vi "main.vi"() -> ()   [LabVIEW 2016]
uses:
  <userlib>/atmcd64d.llb/Error Code Enum typedef.ctl
  <userlib>/atmcd64d.llb/Shutter_mode typedef.ctl
  <vilib>/Utility/miscctls.llb/LVPoint32TypeDef.ctl
  <userlib>/atmcd64d.llb/Shutter_type typedef.ctl
  subVIs/variables/configDB.vi
  subVIs/variables/imageSettings.vi
  subVIs/variables/applicationControl.vi
  subVIs/variables/displayImage.vi
panel:
  in  "left profie location":dbl caption="Wavelength" step=1.0 format="%#.5f"
  in  "right Coords":T1
  in  "Read File":bool
  in  "Read mode":bool
  in  "right wvf scale 3":bool
  in  "left wvf scale 2":bool
  in  "right graph scale 2":bool
  in  "left graph scale":bool
  in  "right wvf color 4":u32(colorbox)=16725034 caption="Marker Color"
  in  "left wvf color 3":u32(colorbox)=16725034 caption="Marker Color"
  in  "left color 2":u32(colorbox)=16725034 caption="Marker Color"
  in  "right color":u32(colorbox)=16725034 caption="Marker Color"
  in  "graph real ratio?":bool caption="Fill screen / Real ratio"
  in  "left Coords":T1
  in  "line avg?":bool
  in  "Line Profile":string(combo)="Horizontal"
  out "scanned?":bool
  in  "right WaveMouse 2":i32
  in  "right Wavelength":dbl caption="Wavelength" step=1.0 format="%#.2f"
  out "Intensity 2":i32 caption="Intensity"
  out "right wvf graph":i32[](graph) caption="On Sensor Image Average"
  in  "left Wavelength":dbl caption="Y (mm)" step=0.01 format="%.2f"
  out "Intensity":i32
  in  "left WaveMouse":i32
  in  "Divide Reference":bool
  in  "Substract Background":bool
  in  "Reference":bool
  in  "Background":bool
  in  "ROI Scan":bool
  in  "ROI":cluster{dbl, dbl}(slide)={143.34131736526948, 408.85429141716565} scale=10.0..535.4
  out "OM":picture
  in  "Exposure Time":u16(ring)=128 items=["1/8000"=160, "1/6400"=157, "1/6000"=156, "1/5000"=155, "1/4000"=152, "1/3200"=149, "1/3000"=148, "1/2500"=147, "1/2000"=144, "1/1600"=141, "1/1500"=140, "1/1250"=139, "1/100"=136, "1/800"=133, "1/640"=131, "1/500"=128, "1/400"=125, "1/320"=123, "1/250"=120, "1/200"=117, "1/160"=115, "1/125"=112, "1/100"=109, "1/80"=107, "1/60"=104, "1/50"=101, "1/40"=99, "1/30"=96, "1/25"=93, "1/8"=80, "1/6"=77, "1/5"=75, "1/4"=72, "0\"3"=69, "0\"4"=67, "0\"5"=64, "0\"6"=61, "0\"7"=60, "0\"8"=59, "1\""=56, "1\"3"=53, "1\"5"=52, "1\"6"=51, "2\""=48, "2\"5"=45, "3\""=44, "3\"2"=43, "4\""=40, "5\""=37, "6\""=35, "8\""=32, "10\""=29, "13\""=27, "15\""=24, "20\""=21, "25\""=19, "30\""=16]
  in  "ISO":u32(ring) items=["Auto"=0, "50"=64, "100"=72, "125"=75, "160"=77, "200"=80, "250"=83, "320"=85, "400"=88, "500"=91, "640"=93, "800"=96, "1000"=99, "1250"=101, "1600"=104, "2000"=107, "2500"=109, "3200"=112, "4000"=115, "5000"=117, "6400"=120, "8000"=123, "10000"=125, "12800"=128, "25600"=136, "51200"=144, "102400"=152, "204800"=160, "409600"=168]
  out "Constructing data":i32(slide) scale=0.0..384.0
  out "Scanning done":bool
  in  "String":string
  in  "Exposure Time:":dbl(slide) scale=1.0..100.0
  out "ET Labelµ":dbl format="%#_3g"
  out "new picture":picture
  in  "Red Gain":i32(slide)=20 scale=1.0..64.0
  in  "Green Gain":i32(slide)=16 scale=1.0..64.0
  in  "Blue Gain":i32(slide)=17 scale=1.0..64.0
  in  "Gain?":bool
  in  "gamma":i32=10 min=1 max=20
  in  "contrast":i32=50 min=0 max=100
  in  "bright":i32=50 min=0 max=100
  in  "sharp":i32 min=0 max=3
  in  "OM":bool
  out "Moving":bool
  in  "Go Origin":bool caption="Origin Return"
  in  "Set Origin":bool
  in  "Stage Position":string
  out "Cooler":bool
  in  "Go back after scan":bool=TRUE
  in  "Scan Step (um)":dbl
  in  "Step length (um)":dbl=100.0
  in  "go left Button":bool
  in  "go right Button":bool
  in  "Y":dbl step=0.01 format="%#_3g"
  in  "X":dbl step=0.01 format="%#_3g"
  in  "Wipe and Quit":bool
  in  "Path":path=path "C:/Users/Administrator/Desktop/test"
  in  "Bandwidth (Frame)":dbl
  in  "Wavelength slide":i32(slide) scale=413.4192199707031..1005.0010375976562
  out "left wvf graph":i32[](graph) caption="On Sensor Image Average"
  out "Right Graph":i32[][](graph) caption="Object Image"
  out "Recovering Temperature":bool
  out "Left Graph":i32[][](graph) caption="On Sensor Image"
  out "temp. status 2":T2
  out "Detector Model":string
  in  "Save File":bool
  in  "Shut Down":bool
  in  "Scan Abort":bool
  out "Current \nScan Frame":dbl
  out "Total \nScan Frame":dbl
  in  "Scan Start":bool
  in  "Scan Length (mm)":dbl=25.0
  in  "Shutter Control":T3=enum."Close"
  in  "Exposure Time (s)":sgl=0.01 step=0.001 format="%.4f"
  in  "Take shot":bool
  in  "VSS (s)":u16(ring)
  in  "HSS (MHz)":i32(ring)
  in  "Live View":bool
  out "Status":T2
  out "Temperature":dbl
  in  "Set Temperature":dbl=20.0
  in  "Initilization File":path=path "C:/Users/Administrator/Desktop/micro.ini"
  # "Image Settings"
  # "Stage Control"
  # "File"
  # "Scan"
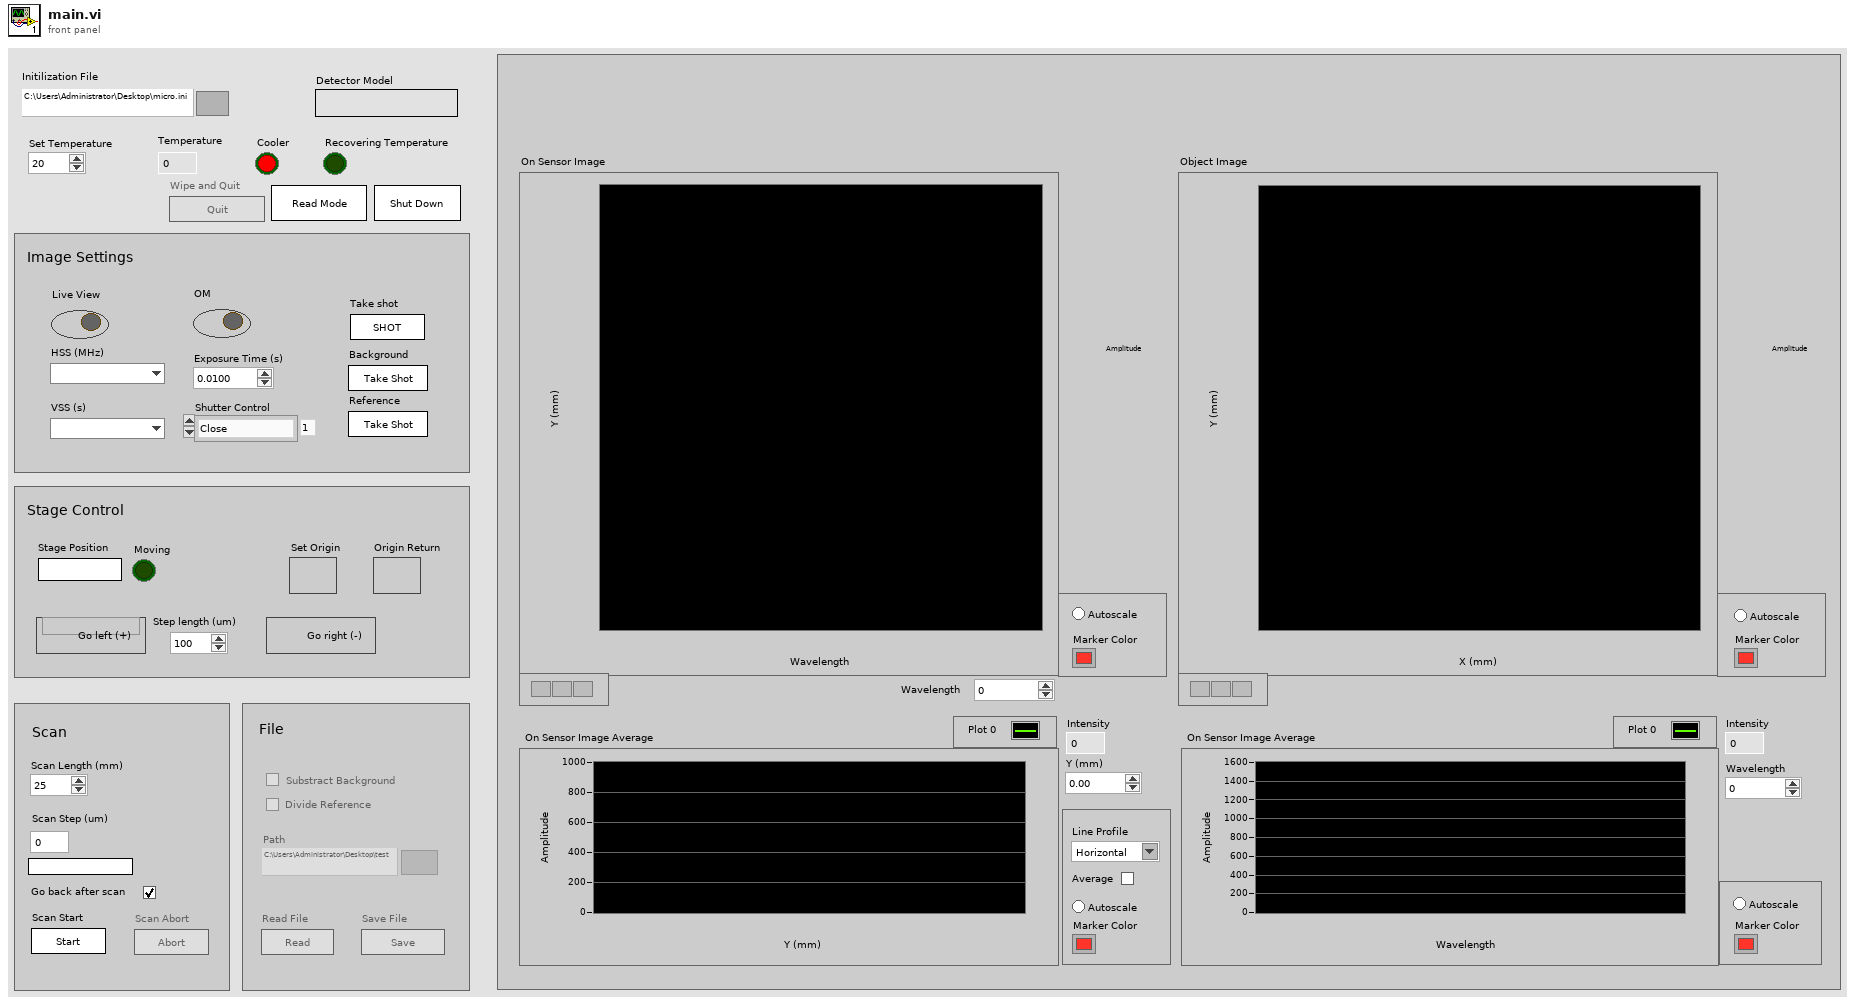
[diagram p1: front panel]
types:
  T1 = typedef "LVPoint32TypeDef.ctl" = cluster{"Horizontal":i32, "Vertical":i32}
  T2 = typedef "Error Code Enum typedef.ctl" = enum32{"N/A (0)", "DRV_ERROR_CODES", "DRV_SUCCESS", "DRV_VXDNOTINSTALLED", "DRV_ERROR_SCAN", "DRV_ERROR_CHECK_SUM", "DRV_ERROR_FILELOAD", "DRV_UNKNOWN_FUNC", "DRV_ERROR_VXD_INIT", "DRV_ERROR_ADDRESS", "DRV_ERROR_PAGELOCK", "DRV_ERROR_PAGEUNLOCK", "DRV_ERROR_BOARDTEST", "DRV_ERROR_ACK", "DRV_ERROR_UP_FIFO", "DRV_ERROR_PATTERN", "N/A (16)", "DRV_ACQUISITION_ERRORS", "DRV_ACQ_BUFFER", "DRV_ACQ_DOWNFIFO_FULL", "DRV_PROC_UNKONWN_INSTRUCTION", "DRV_ILLEGAL_OP_CODE", "DRV_KINETIC_TIME_NOT_MET", "DRV_ACCUM_TIME_NOT_MET", "DRV_NO_NEW_DATA", "N/A (25)", "DRV_SPOOLERROR", "N/A (27)", "N/A (28)", "N/A (29)", "N/A (30)", "N/A (31)", "N/A (32)", "DRV_TEMPERATURE_CODES", "DRV_TEMPERATURE_OFF", "DRV_TEMPERATURE_NOT_STABILIZED", "DRV_TEMPERATURE_STABILIZED", "DRV_TEMPERATURE_NOT_REACHED", "DRV_TEMPERATURE_OUT_RANGE", "DRV_TEMPERATURE_NOT_SUPPORTED", "DRV_TEMPERATURE_DRIFT", "N/A (41)", "N/A (42)", "N/A (43)", "N/A (44)", "N/A (45)", "N/A (46)", "N/A (47)", "N/A (48)", "DRV_GENERAL_ERRORS", "DRV_INVALID_AUX", "DRV_COF_NOTLOADED", "DRV_FPGAPROG", "DRV_FLEXERROR", "DRV_GPIBERROR", "N/A (55)", "N/A (56)", "N/A (57)", "N/A (58)", "N/A (59)", "N/A (60)", "N/A (61)", "N/A (62)", "N/A (63)", "DRV_DATATYPE", "DRV_DRIVER_ERRORS", "DRV_P1INVALID", "DRV_P2INVALID", "DRV_P3INVALID", "DRV_P4INVALID", "DRV_INIERROR", "DRV_COFERROR", "DRV_ACQUIRING", "DRV_IDLE", "DRV_TEMPCYCLE", "DRV_NOT_INITIALIZED", "DRV_P5INVALID", "DRV_P6INVALID", "DRV_INVALID_MODE", "DRV_INVALID_FILTER", "DRV_I2CERRORS", "DRV_I2CDEVNOTFOUND", "DRV_I2CTIMEOUT", "DRV_P7INVALID", "N/A (84)", "N/A (85)", "N/A (86)", "N/A (87)", "N/A (88)", "N/A (89)", "DRV_IOCERROR", "DRV_VRMVERSIONERROR"}
  T3 = typedef "Shutter_mode typedef.ctl" = enum16{"Auto", "Close", "Open", "N/A (3)", "Open FVB Series", "Open Any Series"}
  T4 = enum8{"Enabled", "Disabled", "Disabled and Grayed Out"}
  T5 = cluster{"Width":u16, "Style":enum32{"Solid", "Dash", "Dot", "DashDot", "DashDotDot"}}
  T6 = typedef "Shutter_type typedef.ctl" = enum16{"TTL Low", "TTL High"}
  T7 = typedef "HSSpeed_type typedef.ctl" = enum16{"EM Amp", "Conventional Amp"}
  T8 = typedef "LVMouseTypeDef.ctl" = cluster{"Mouse Position":cluster{"X":i32, "Y":i32}, "Mouse Modifiers":cluster{"Button Down":bool, "Shift Mod":bool, "Menu Mod":bool, "Option Mod":bool}}
  T9 = typedef "imagedata.ctl" = cluster{"image type":i32, "image depth":i32, "image":u8[], "mask":u8[], "colors":u32[], "Rectangle":cluster{"left":i16, "top":i16, "right":i16, "bottom":i16}}
  T10 = typedef "LVBoundsTypeDef.ctl" = cluster{"Width":u32, "Height":u32}
  T11 = cluster{"left":i16, "top":i16, "right":i16, "bottom":i16}
  T12 = cluster{"Scan Abort":refnum<vi>, "Constructing data":refnum<vi>, "Right Graph":refnum<vi>, "Left Graph":refnum<vi>, "Total \nScan Frame":refnum<vi>, "Current \nScan Frame":refnum<vi>}
  T13 = typedef "LVRectTypeDef.ctl" = cluster{"Left":i16, "Top":i16, "Right":i16, "Bottom":i16}
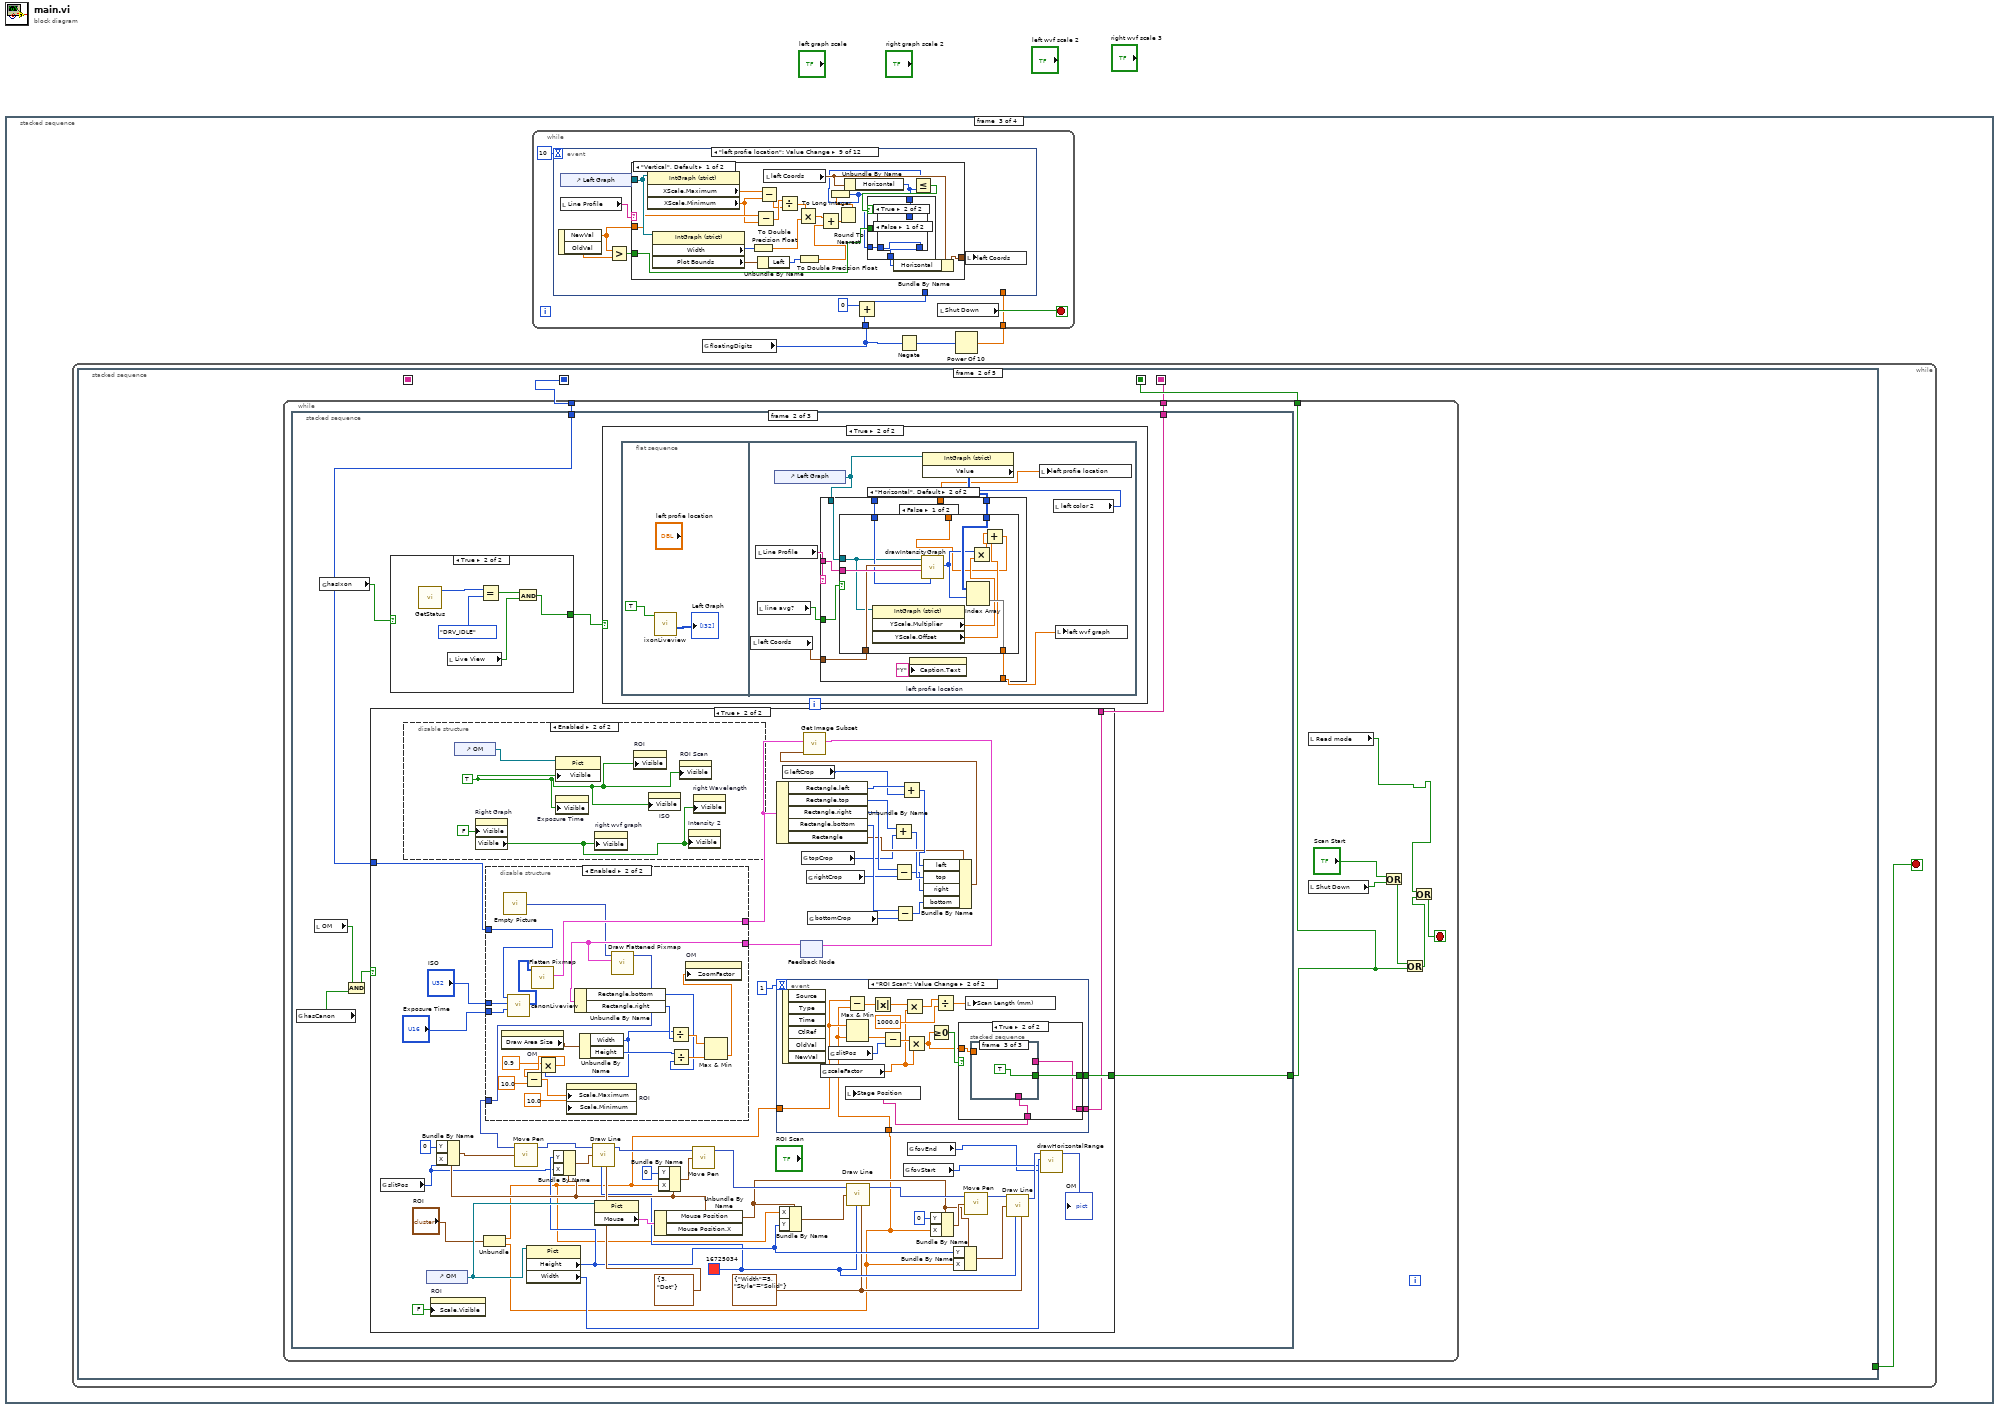
[diagram p0: block diagram]
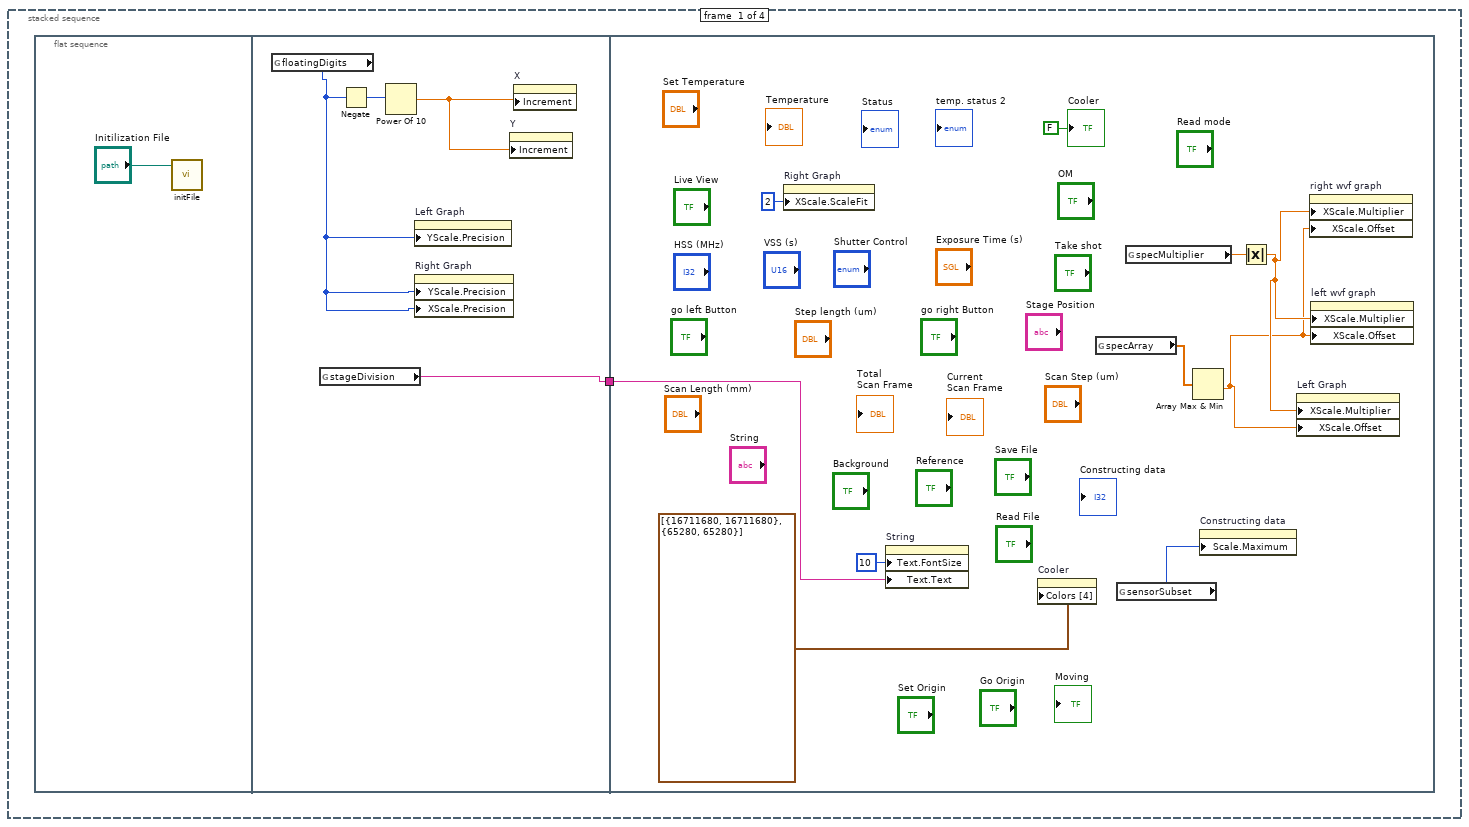
[diagram p2: hidden frame]
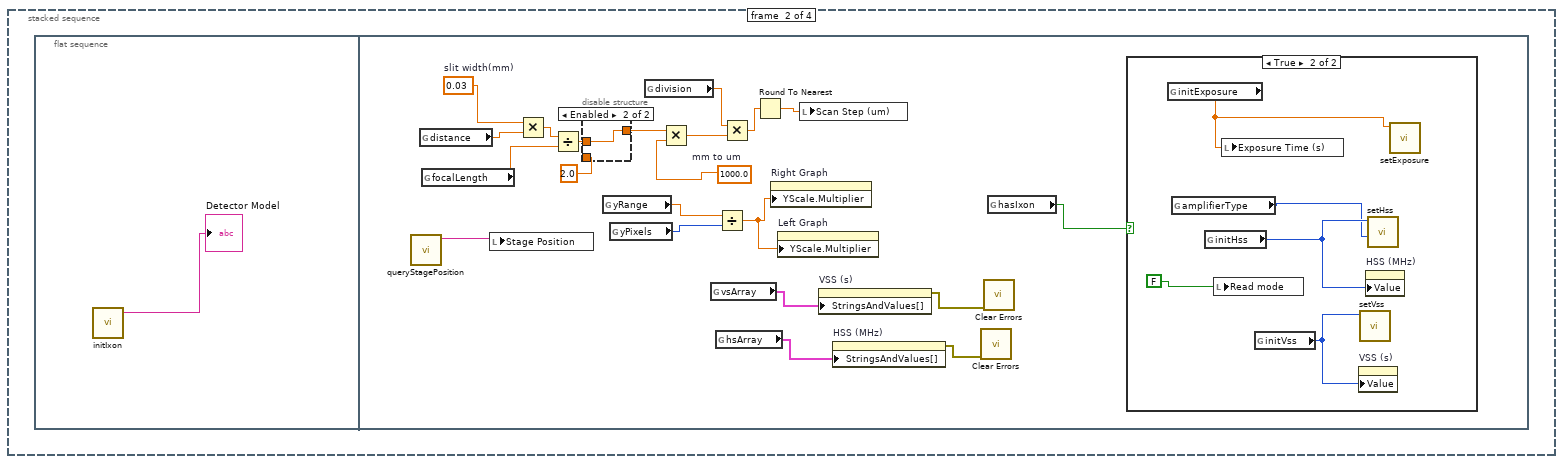
[diagram p3: hidden frame]
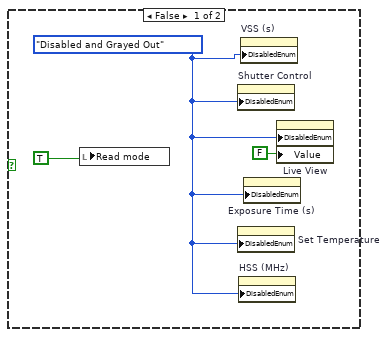
[diagram p4: hidden frame]
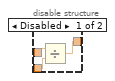
[diagram p5: hidden frame]
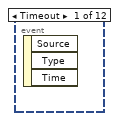
[diagram p6: hidden frame]
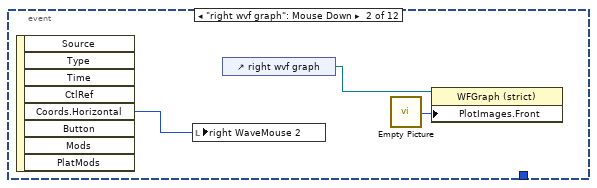
[diagram p7: hidden frame]
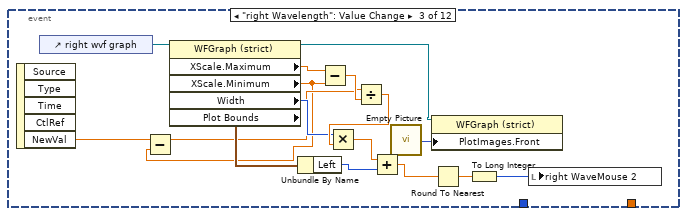
[diagram p8: hidden frame]
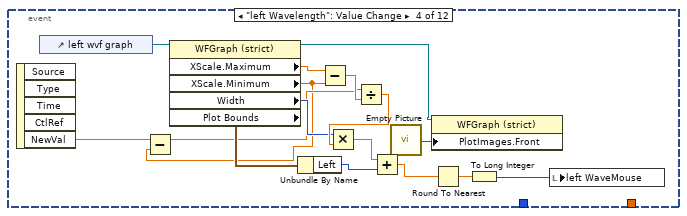
[diagram p9: hidden frame]
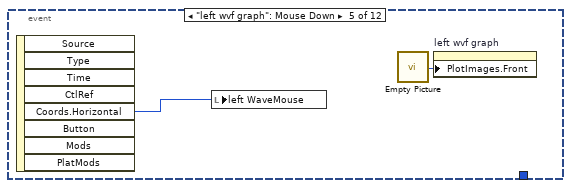
[diagram p10: hidden frame]
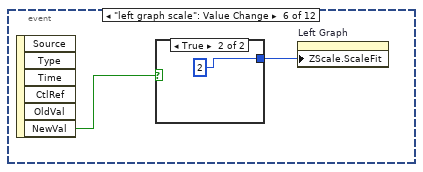
[diagram p11: hidden frame]
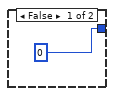
[diagram p12: hidden frame]
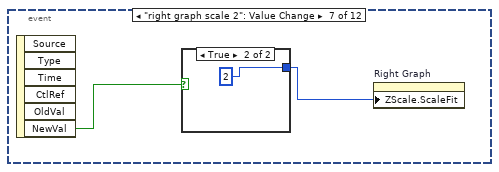
[diagram p13: hidden frame]
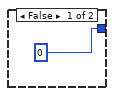
[diagram p14: hidden frame]
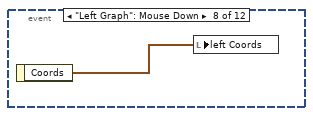
[diagram p15: hidden frame]
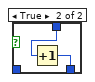
[diagram p17: hidden frame]
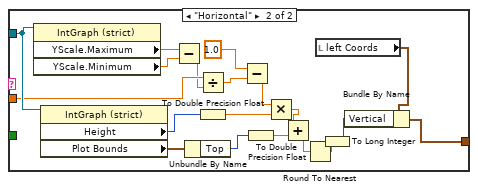
[diagram p18: hidden frame]
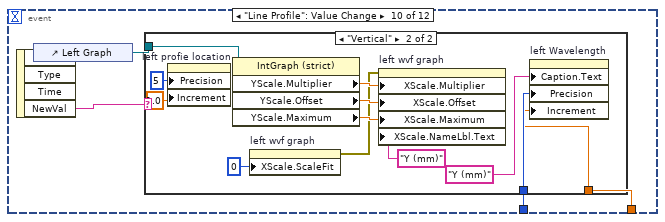
[diagram p19: hidden frame]
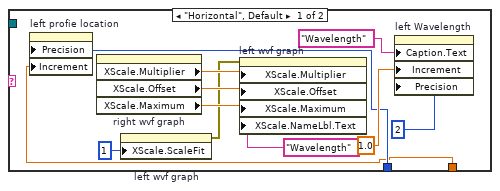
[diagram p20: hidden frame]
diagram:
  n1 = stacked-sequence {
    frame #0 {
      n2 = flat-sequence {
        tunnel: [w6] -> w1
        tunnel: w1 -> [w13]
        frame #0 {
          n3 = call "initFile.vi"("Init File"="Initilization File") -> ()  [unwired: 11 in]
        }
        frame #1 {
          n4 = global read "configDB.vi" "floatingDigits"() -> (w5:i32)
          n5 = global read "configDB.vi" "stageDivision"() -> (w6:string)
          n6 = Negate(x=w5) -> (-x=w4:i32)
          n7 = Power Of 10(x=w4) -> (10^x=w3:dbl)
          n8 = property on="Left Graph" class="IntGraph (strict)"("YScale.Precision"=w5) -> ()  [unwired: 2 in, 2 out]
          n9 = property on="Right Graph" class="IntGraph (strict)"("YScale.Precision"=w5, "XScale.Precision"=w5) -> ()  [unwired: 2 in, 2 out]
          n10 = property on="Y" class="DigNum (strict)"("Increment"=w3) -> ()  [unwired: 2 in, 2 out]
          n11 = property on="X" class="DigNum (strict)"("Increment"=w3) -> ()  [unwired: 2 in, 2 out]
        }
        frame #2 {
          n12 = property on="Right Graph" class="IntGraph (strict)"("XScale.ScaleFit"=u8 2 ("X Scale.Scale Fit")) -> ()  [unwired: 2 in, 2 out]
          n13 = property on="String" class="Str"("Text.FontSize"=u32 10 ("Text.Font:Size"), "Text.Text"=w13) -> ()  [unwired: 2 in, 2 out]
          n14 = property on="Cooler" class="Bool (strict)"("Colors [4]"=cluster{u32, u32}[] [{16711680, 16711680}, {65280, 65280}]) -> ()  [unwired: 2 in, 2 out]
          n15 = global read "imageSettings.vi" "specArray"() -> (w10:sgl[])
          n16 = global read "configDB.vi" "sensorSubset"() -> (w7:i32)
          n17 = global read "configDB.vi" "specMultiplier"() -> (w11:dbl)
          n18 = Array Max & Min(array=w10) -> (min value=w8:sgl)  [unwired: 3 out]
          n19 = property on="Constructing data" class="Slide (strict)"("Scale.Maximum"=w7) -> ()  [unwired: 2 in, 2 out]
          n20 = Absolute Value(x=w11) -> (abs(x)=w9:dbl)
          n21 = property on="Left Graph" class="IntGraph (strict)"("XScale.Multiplier"=w9, "XScale.Offset"=w8) -> ()  [unwired: 2 in, 2 out]
          n22 = property on="right wvf graph" class="WFGraph (strict)"("XScale.Multiplier"=w9, "XScale.Offset"=w8) -> ()  [unwired: 2 in, 2 out]
          n23 = property on="left wvf graph" class="WFGraph (strict)"("XScale.Multiplier"=w9, "XScale.Offset"=w8) -> ()  [unwired: 2 in, 2 out]
          "Cooler" <- FALSE ("Cooler")
        }
      }
    }
    frame #1 {
      n24 = flat-sequence {
        frame #0 {
          n25 = call "initIxon.vi"() -> ("model"=→"Detector Model":string)  [unwired: 5 in, 2 out]
        }
        frame #1 {
          w30 = 1000.0  # mm to um
          w37 = 0.03  # slit width(mm)
          n26 = call "queryStagePosition.vi"() -> ("stagePosition"=w28:string)  [unwired: 11 in]
          n27 = global read "configDB.vi" "distance"() -> (w26:dbl)
          n28 = global read "configDB.vi" "focalLength"() -> (w25:dbl)
          n29 = local write "Stage Position"(w28) -> ()
          n30 = Multiply(x=w37, y=w26) -> (x*y=w36:dbl)
          n31 = Divide(x=w36, y=w25) -> (x/y=w34:dbl)
          n32 = disable-structure shown="Enabled" {
            disable-tunnel: w34 -> [w49 w50]
            disable-tunnel: 2.0 ("y") -> [w48 _]
            disable-tunnel: [w47 w50] -> w32
            frame Disabled {
              n33 = Divide(x=w49, y=w48) -> (x/y=w47:dbl)
            }
            frame Enabled {
            }
          }
          n34 = global read "configDB.vi" "yRange"() -> (w24:dbl)
          n35 = global read "configDB.vi" "yPixels"() -> (w19:i32)
          n36 = global read "configDB.vi" "division"() -> (w27:dbl)
          n37 = Multiply(x=w32, y=w30) -> (x*y=w35:dbl)
          n38 = global read "imageSettings.vi" "vsArray"() -> (w22:cluster{"String":string, "Value":u16}[])
          n39 = global read "imageSettings.vi" "hsArray"() -> (w23:cluster{"String":string, "Value":u16}[])
          n40 = Divide(x=w24, y=w19) -> (x/y=w38:dbl)
          n41 = Multiply(x=w27, y=w35) -> (x*y=w31:dbl)
          n42 = Round To Nearest(number=w31) -> (nearest integer value=w29:dbl)
          n43 = property on="Right Graph" class="IntGraph (strict)"("YScale.Multiplier"=w38) -> ()  [unwired: 2 in, 2 out]
          n44 = property on="Left Graph" class="IntGraph (strict)"("YScale.Multiplier"=w38) -> ()  [unwired: 2 in, 2 out]
          n45 = local write "Scan Step (um)"(w29) -> ()
          n46 = property on="VSS (s)" class="Ring (strict)"("StringsAndValues[]"=w22) -> (error out=w21:errorcluster)  [unwired: 2 in, 1 out]
          n47 = property on="HSS (MHz)" class="Ring (strict)"("StringsAndValues[]"=w23) -> (error out=w20:errorcluster)  [unwired: 2 in, 1 out]
          n48 = call <vilib>:"Clear Errors.vi"("error in (no error)"=w20) -> ()  [unwired: 5 in, 2 out]
          n49 = call <vilib>:"Clear Errors.vi"("error in (no error)"=w21) -> ()  [unwired: 5 in, 2 out]
          n50 = global read "applicationControl.vi" "hasIxon"() -> (w18:bool)
          n51 = case shown="True" w18 {
            frame False {
              w41 = T4."Disabled and Grayed Out" ("Disabled")
              n52 = local write "Read mode"(TRUE) -> ()
              n53 = property on="Shutter Control" class="Enum (strict)"("DisabledEnum"=w41) -> ()  [unwired: 2 in, 2 out]
              n54 = property on="Set Temperature" class="DigNum (strict)"("DisabledEnum"=w41) -> ()  [unwired: 2 in, 2 out]
              n55 = property on="HSS (MHz)" class="Ring (strict)"("DisabledEnum"=w41) -> ()  [unwired: 2 in, 2 out]
              n56 = property on="VSS (s)" class="Ring (strict)"("DisabledEnum"=w41) -> ()  [unwired: 2 in, 2 out]
              n57 = property on="Exposure Time (s)" class="DigNum (strict)"("DisabledEnum"=w41) -> ()  [unwired: 2 in, 2 out]
              n58 = property on="Live View" class="Bool (strict)"("DisabledEnum"=w41, "Value"=FALSE ("Live View")) -> ()  [unwired: 2 in, 2 out]
            }
            frame True {
              n59 = global read "configDB.vi" "initExposure"() -> (w46:dbl)
              n60 = global read "configDB.vi" "amplifierType"() -> (w43:T7)
              n61 = global read "configDB.vi" "initHss"() -> (w45:i32)
              n62 = local write "Read mode"(FALSE) -> ()
              n63 = local write "Exposure Time (s)"(w46) -> ()
              n64 = global read "configDB.vi" "initVss"() -> (w44:i32)
              n65 = property on="VSS (s)" class="Ring (strict)"("Value"=w44) -> ()  [unwired: 2 in, 2 out]
              n66 = call "setVss.vi"("index"=w44) -> ()  [unwired: 11 in]
              n67 = property on="HSS (MHz)" class="Ring (strict)"("Value"=w45) -> ()  [unwired: 2 in, 2 out]
              n68 = call "setHss.vi"("type"=w43, "index"=w45) -> ()  [unwired: 10 in]
              n69 = call "setExposure.vi"("Exposure Time (s)"=w46) -> ()  [unwired: 11 in]
            }
          }
        }
      }
    }
    frame #2 {
      n70 = while {
        stop <- w196 stop-if-true
        n71 = stacked-sequence {
          seq-local: [_ _ w535 _ _] -> [_ _ _ w565 _]
          seq-local: [w199 _ _ _ _] -> [_ w213 w534 _ _]
          seq-local: [_ w212 _ _ _] -> [_ _ _ w567 _]
          seq-local: [_ w211 _ _ _] -> [_ _ _ w566 _]
          tunnel: [_ _ _ _ w603] -> w196
          frame #0 {
            n72 = flat-sequence {
              tunnel: [w202] -> w199
              tunnel: [w201] -> w197
              tunnel: [w206] -> w198
              tunnel: w197 -> [w206]
              tunnel: w198 -> [w210]
              frame #0 {
                n73 = disable-structure shown="Enabled" {
                  disable-tunnel: [_ w205] -> w202
                  disable-tunnel: [_ w204] -> w201
                  frame Disabled {
                    n74 = call "initMightex.vi"() -> ()  [unwired: 11 in, 1 out]
                  }
                  frame Enabled {
                    n75 = call "initCanon.vi"() -> ("error out"=w203:errorcluster, "inRef dup"=w205:u32)  [unwired: 10 in]
                    n76 = Unbundle By Name(w203) -> ("status"=w204:bool)
                    n77 = call <vilib>:"Clear Errors.vi"("error in (no error)"=w203) -> ()  [unwired: 5 in, 2 out]
                  }
                }
              }
              frame #1 {
                n78 = global read "applicationControl.vi" "hasCanon"() -> (w207:bool)
                n79 = case shown="False" w207 {
                  frame False {
                    n80 = property on="OM" class="Bool (strict)"("DisabledEnum"=T4."Disabled and Grayed Out" ("Disabled"), "Value"=FALSE ("OM")) -> ()  [unwired: 2 in, 2 out]
                  }
                  frame True {
                  }
                }
              }
              frame #2 {
                n81 = case shown="True" w210 {
                  frame False {
                  }
                  frame True {
                    n82 = call "Display Message to User"() -> ()  [unwired: 10 in, 2 out]
                  }
                }
              }
            }
            n83 = call "queryStagePosition.vi"() -> ("stagePosition"=w200:string)  [unwired: 11 in]
            n84 = local write "Stage Position"(w200) -> ()
          }
          frame #1 {
            n85 = while {
              tunnel: w213 -> [w220]
              tunnel: [w218] -> w212
              tunnel: [w217] -> w211
              stop <- w215 stop-if-true
              n86 = stacked-sequence {
                tunnel: w220 -> [_ w288 _]
                tunnel: [_ w287 _] -> w218
                tunnel: [_ w286 _] -> w217
                frame #0 {
                  n87 = event shown="[3] \"Background\": Value Change" {
                    selector: _ -> [_ _ _ _ _ _ _ _ _ _ _ _ _ _]
                    dyn-events: _ -> [_ _ _ _ _ _ _ _ _ _ _ _ _ _]
                    timeout: 0 -> [_ _ _ _ _ _ _ _ _ _ _ _ _ _]
                    event "HSS (MHz)": Value Change {
                      n88 = event-data() -> ()  [unwired: 1 in, 6 out]
                      n89 = global read "configDB.vi" "amplifierType"() -> (w227:T7)
                      n90 = property on="HSS (MHz)" class="Ring (strict)"() -> ("Value"=w228:i32)  [unwired: 2 in, 2 out]
                      n91 = call "setHss.vi"("type"=w227, "index"=w228) -> ()  [unwired: 10 in]
                    }
                    event "VSS (s)": Value Change {
                      n92 = event-data() -> ()  [unwired: 1 in, 6 out]
                      n93 = property on="VSS (s)" class="Ring (strict)"() -> ("Value"=w229:u16)  [unwired: 2 in, 2 out]
                      n94 = call "setVss.vi"("index"=w229) -> ()  [unwired: 11 in]
                    }
                    event "Take shot": Value Change {
                      n95 = event-data() -> ()  [unwired: 1 in, 6 out]
                      n96 = flat-sequence {
                        frame #0 {
                          n97 = global read "configDB.vi" "specMultiplier"() -> (w233:dbl)
                          n98 = global read "imageSettings.vi" "specArray"() -> (w231:sgl[])
                          n99 = Array Max & Min(array=w231) -> (min value=w230:sgl)  [unwired: 3 out]
                          n100 = Absolute Value(x=w233) -> (abs(x)=w232:dbl)
                          n101 = property on="Right Graph" class="IntGraph (strict)"("XScale.Multiplier"=w232, "XScale.Offset"=w230, "XScale.NameLbl.Text"="Wavelength (nm)" ("X Scale.Name Label.Text"), "Caption.Text"="On Sensor Image" ("Label.Text")) -> ()  [unwired: 2 in, 2 out]
                        }
                        frame #1 {
                          n102 = call "ixonLiveview.vi"("stop"=TRUE) -> ("Left Graph"=→"Right Graph":i32[][])  [unwired: 10 in]
                        }
                        frame #2 {
                          n103 = control-ref of="Right Graph"() -> (w239:refnum<vi>)
                          n104 = property on="Property Node" class="IntGraph (strict)"(reference=w239) -> ("Value"=w238:i32[][])  [unwired: 1 in, 2 out]
                          n105 = for {
                            N: 384 -> [_]
                            tunnel: w238 -> [w247]
                            tunnel: [w242] -> w241 mode=indexing
                            i -> [w246]
                            n106 = Index Array(array=w247, index (col)=w246) -> (element=w245:i32[])  [unwired: 1 in]
                            n107 = Add Array Elements(numeric array=w245) -> (sum=w244:i32)
                            n108 = Divide(x=w244, y=512) -> (x/y=w242:dbl)
                          }
                          n109 = local write "right wvf graph"(w241) -> ()
                        }
                      }
                    }
                    event "Background": Value Change {
                      n110 = event-data() -> ()  [unwired: 1 in, 6 out]
                      n111 = flat-sequence {
                        frame #0 {
                          n112 = call "setShutterMode.vi"("mode"=Shutter_mode_typedef."Close") -> ()  [unwired: 11 in]
                        }
                        frame #1 {
                          n113 = Wait (ms)(milliseconds to wait=u32 1000) -> ()  [unwired: 1 out]
                        }
                        frame #2 {
                          n114 = call "ixonLiveview.vi"("stop"=TRUE) -> ("Left Graph"=w250:i32[][])  [unwired: 10 in]
                          n115 = global write "imageSettings.vi" "backgroundExist"(TRUE ("backgroundExist")) -> ()
                          n116 = local write "Right Graph"(w250) -> ()
                          n117 = call "background.vi"("Enum"=enum16{"clear", "read", "write"}."write", "backgroundImageIn"=w250) -> ()  [unwired: 9 in, 1 out]
                        }
                        frame #3 {
                          n118 = local read "Shutter Control"() -> (w254:T3)
                          n119 = call "setShutterMode.vi"("mode"=w254) -> ()  [unwired: 11 in]
                        }
                      }
                    }
                    event "Reference": Value Change {
                      n120 = event-data() -> ()  [unwired: 1 in, 6 out]
                      n121 = flat-sequence {
                        frame #0 {
                          n122 = call "setShutterMode.vi"("mode"=Shutter_mode_typedef."Open") -> ()  [unwired: 11 in]
                        }
                        frame #1 {
                          n123 = Wait (ms)(milliseconds to wait=u32 1000) -> ()  [unwired: 1 out]
                        }
                        frame #2 {
                          n124 = call "ixonLiveview.vi"("stop"=TRUE) -> ("Left Graph"=w257:i32[][])  [unwired: 10 in]
                          n125 = local write "Right Graph"(w257) -> ()
                          n126 = global write "imageSettings.vi" "referenceExist"(TRUE ("backgroundExist")) -> ()
                          n127 = call "reference.vi"("Enum"=enum16{"clear", "read", "write"}."write", "referenceImageIn"=w257) -> ()  [unwired: 9 in, 1 out]
                        }
                        frame #3 {
                          n128 = local read "Shutter Control"() -> (w261:T3)
                          n129 = call "setShutterMode.vi"("mode"=w261) -> ()  [unwired: 11 in]
                        }
                      }
                    }
                    event "go right Button": Value Change {
                      n130 = event-data() -> ()  [unwired: 1 in, 6 out]
                      n131 = flat-sequence {
                        frame #0 {
                          n132 = local write "Moving"(TRUE ("Moving")) -> ()
                        }
                        frame #1 {
                          n133 = local read "Step length (um)"() -> (w264:dbl)
                          n134 = call "stageGoRight.vi"("Step length (um)"=w264) -> ("Stage Position"=w263:string)  [unwired: 10 in]
                          n135 = local write "Stage Position"(w263) -> ()
                        }
                        frame #2 {
                          n136 = local write "Moving"(FALSE ("Moving")) -> ()
                        }
                      }
                    }
                    event "Go Origin": Value Change {
                      n137 = event-data() -> ()  [unwired: 1 in, 6 out]
                      n138 = flat-sequence {
                        frame #0 {
                          n139 = local write "Moving"(TRUE ("Moving")) -> ()
                        }
                        frame #1 {
                          n140 = call "stageGoOrigin.vi"() -> ()  [unwired: 12 in]
                        }
                        frame #2 {
                          n141 = local write "Stage Position"("0" ("Stage Position")) -> ()
                          n142 = local write "Moving"(FALSE ("Moving")) -> ()
                        }
                      }
                    }
                    event "Set Origin": Value Change {
                      n143 = event-data() -> ()  [unwired: 1 in, 6 out]
                      n144 = local write "Stage Position"("0" ("Stage Position")) -> ()
                      n145 = call "stageSetOrigin.vi"() -> ()  [unwired: 12 in]
                    }
                    event "go left Button": Value Change {
                      n146 = event-data() -> ()  [unwired: 1 in, 6 out]
                      n147 = flat-sequence {
                        frame #0 {
                          n148 = local write "Moving"(TRUE ("Moving")) -> ()
                        }
                        frame #1 {
                          n149 = local read "Step length (um)"() -> (w272:dbl)
                          n150 = call "stageGoLeft.vi"("Step length (um)"=w272) -> ("Stage Position"=w271:string)  [unwired: 10 in]
                          n151 = local write "Stage Position"(w271) -> ()
                        }
                        frame #2 {
                          n152 = local write "Moving"(FALSE ("Moving")) -> ()
                        }
                      }
                    }
                    event "Scan Step (um)": Value Change {
                      n153 = event-data() -> ()  [unwired: 1 in, 6 out]
                      n154 = local read "Scan Step (um)"() -> (w275:dbl)
                      n155 = global read "configDB.vi" "division"() -> (w274:dbl)
                      n156 = Quotient & Remainder(x=w275, y=w274) -> (x-y*floor(x/y)=w278:dbl)  [unwired: 1 out]
                      n157 = Equal?(x=w278, y=0.0) -> (x = y?=w276:bool)
                      n158 = case shown="False" w276 {
                        frame False {
                          n159 = call "Step too small!"() -> ()  [unwired: 18 in, 2 out]
                        }
                        frame True {
                        }
                      }
                    }
                    event Timeout {
                      n160 = event-data() -> ()  [unwired: 1 in, 3 out]
                    }
                    event Value Change {
                      n161 = event-data() -> ()  [unwired: 1 in, 6 out]
                      n162 = property on="Shutter Control" class="Enum (strict)"() -> ("Value"=w279:T3)  [unwired: 2 in, 2 out]
                      n163 = call "setShutterMode.vi"("mode"=w279) -> ()  [unwired: 11 in]
                    }
                    event "Exposure Time (s)": Value Change {
                      n164 = event-data() -> ()  [unwired: 1 in, 6 out]
                      n165 = local read "Exposure Time (s)"() -> (w280:sgl)
                      n166 = call "setExposure.vi"("Exposure Time (s)"=w280) -> ()  [unwired: 11 in]
                    }
                    event "Set Temperature": Value Change {
                      n167 = event-data() -> ()  [unwired: 1 in, 6 out]
                      n168 = local read "Set Temperature"() -> (w281:dbl)
                      n169 = call "setTemp.vi"("Set Temp."=w281) -> ()  [unwired: 11 in]
                    }
                  }
                  n170 = global read "imageSettings.vi" "backgroundExist"() -> (w223:bool)
                  n171 = case shown="True" w223 {
                    frame False {
                      n172 = property on="Reference" class="Bool"("DisabledEnum"=T4."Disabled and Grayed Out" ("Disabled")) -> ()  [unwired: 2 in, 2 out]
                    }
                    frame True {
                      n173 = property on="Reference" class="Bool"("DisabledEnum"=T4."Enabled" ("Disabled")) -> ()  [unwired: 2 in, 2 out]
                    }
                  }
                }
                frame #1 {
                  n174 = global read "applicationControl.vi" "hasCanon"() -> (w283:bool)
                  n175 = local read "OM"() -> (w284:bool)
                  n176 = global read "applicationControl.vi" "hasIxon"() -> (w282:bool)
                  n177 = And(x=w284, y=w283) -> (x .and. y?=w285:bool)
                  n178 = case shown="True" w285 {
                    tunnel: w288 -> [_ w432]
                    tunnel: [FALSE w389] -> w287
                    tunnel: [_ w385] -> w286
                    frame False {
                      w373 = FALSE ("Visible")
                      w377 = FALSE ("Visible")
                      n179 = property on="new picture" class="Pict"("Visible"=w377) -> ()  [unwired: 2 in, 2 out]
                      n180 = property on="sharp" class="DigNum (strict)"("Visible"=w377) -> ()  [unwired: 2 in, 2 out]
                      n181 = property on="bright" class="DigNum (strict)"("Visible"=w377) -> ()  [unwired: 2 in, 2 out]
                      n182 = property on="gamma" class="DigNum (strict)"("Visible"=w377) -> ()  [unwired: 2 in, 2 out]
                      n183 = property on="Exposure Time:" class="Slide (strict)"("Visible"=w377) -> ()  [unwired: 2 in, 2 out]
                      n184 = property on="ET Labelµ" class="DigNum (strict)"("Visible"=w377) -> ()  [unwired: 2 in, 2 out]
                      n185 = property on="Right Graph" class="IntGraph (strict)"("Visible"=TRUE) -> ("Visible"=w370:bool)  [unwired: 2 in, 2 out]
                      n186 = property on="right wvf graph" class="WFGraph (strict)"("Visible"=w370) -> ()  [unwired: 2 in, 2 out]
                      n187 = property on="right Wavelength" class="DigNum (strict)"("Visible"=w370) -> ()  [unwired: 2 in, 2 out]
                      n188 = property on="Intensity 2" class="DigNum (strict)"("Visible"=w370) -> ()  [unwired: 2 in, 2 out]
                      n189 = property on="contrast" class="DigNum (strict)"("Visible"=w377) -> ()  [unwired: 2 in, 2 out]
                      n190 = property on="Red Gain" class="Slide (strict)"("Visible"=w377) -> ()  [unwired: 2 in, 2 out]
                      n191 = property on="Blue Gain" class="Slide (strict)"("Visible"=w377) -> ()  [unwired: 2 in, 2 out]
                      n192 = property on="Green Gain" class="Slide (strict)"("Visible"=w377) -> ()  [unwired: 2 in, 2 out]
                      n193 = property on="Gain?" class="Bool (strict)"("Visible"=w377) -> ()  [unwired: 2 in, 2 out]
                      n194 = control-ref of="Exposure Time"() -> (w374:refnum<vi>)
                      n195 = control-ref of="OM"() -> (w376:refnum<vi>)
                      n196 = property on="Property Node" class="Ring (strict)"(reference=w374, "Visible"=w373) -> ()  [unwired: 1 in, 2 out]
                      n197 = property on="ROI Scan" class="Bool"("Visible"=w373) -> ()  [unwired: 2 in, 2 out]
                      n198 = control-ref of="ISO"() -> (w375:refnum<vi>)
                      n199 = property on="ROI" class="Slide (strict)"("Visible"=w373) -> ()  [unwired: 2 in, 2 out]
                      n200 = property on="Property Node" class="Pict"(reference=w376, "Visible"=w373) -> ()  [unwired: 1 in, 2 out]
                      n201 = property on="Property Node" class="Ring (strict)"(reference=w375, "Visible"=w373) -> ()  [unwired: 1 in, 2 out]
                    }
                    frame True {
                      w396 = T5 {"Width"=5, "Style"=enum."Solid"} ("pen")
                      w397 = u32 16725034 ("color(black)")
                      n202 = global read "configDB.vi" "slitPos"() -> (w384:i32)
                      n203 = disable-structure shown="Enabled" {
                        frame Disabled {
                          w466 = TRUE ("Visible")
                          n204 = property on="contrast" class="DigNum (strict)"("Visible"=w466) -> ()  [unwired: 2 in, 2 out]
                          n205 = property on="bright" class="DigNum (strict)"("Visible"=w466) -> ()  [unwired: 2 in, 2 out]
                          n206 = property on="sharp" class="DigNum (strict)"("Visible"=w466) -> ()  [unwired: 2 in, 2 out]
                          n207 = property on="gamma" class="DigNum (strict)"("Visible"=w466) -> ()  [unwired: 2 in, 2 out]
                          n208 = property on="new picture" class="Pict"("Visible"=w466) -> ()  [unwired: 2 in, 2 out]
                          n209 = property on="Gain?" class="Bool (strict)"("Visible"=w466) -> ()  [unwired: 2 in, 2 out]
                          n210 = property on="Green Gain" class="Slide (strict)"("Visible"=w466) -> ()  [unwired: 2 in, 2 out]
                          n211 = property on="Red Gain" class="Slide (strict)"("Visible"=w466) -> ()  [unwired: 2 in, 2 out]
                          n212 = property on="Blue Gain" class="Slide (strict)"("Visible"=w466) -> ()  [unwired: 2 in, 2 out]
                          n213 = property on="Exposure Time:" class="Slide (strict)"("Visible"=w466) -> ()  [unwired: 2 in, 2 out]
                          n214 = property on="ET Labelµ" class="DigNum (strict)"("Visible"=w466) -> ()  [unwired: 2 in, 2 out]
                        }
                        frame Enabled {
                          w469 = TRUE ("Visible")
                          n215 = control-ref of="OM"() -> (w470:refnum<vi>)
                          n216 = property on="Right Graph" class="IntGraph (strict)"("Visible"=FALSE) -> ("Visible"=w467:bool)  [unwired: 2 in, 2 out]
                          n217 = property on="Property Node" class="Pict"(reference=w470, "Visible"=w469) -> ()  [unwired: 1 in, 2 out]
                          n218 = property on="Exposure Time" class="Ring (strict)"("Visible"=w469) -> ()  [unwired: 2 in, 2 out]
                          n219 = property on="right wvf graph" class="WFGraph (strict)"("Visible"=w467) -> ()  [unwired: 2 in, 2 out]
                          n220 = property on="ROI" class="Slide (strict)"("Visible"=w469) -> ()  [unwired: 2 in, 2 out]
                          n221 = property on="ISO" class="Ring (strict)"("Visible"=w469) -> ()  [unwired: 2 in, 2 out]
                          n222 = property on="ROI Scan" class="Bool"("Visible"=w469) -> ()  [unwired: 2 in, 2 out]
                          n223 = property on="Intensity 2" class="DigNum (strict)"("Visible"=w467) -> ()  [unwired: 2 in, 2 out]
                          n224 = property on="right Wavelength" class="DigNum (strict)"("Visible"=w467) -> ()  [unwired: 2 in, 2 out]
                        }
                      }
                      n225 = control-ref of="OM"() -> (w419:refnum<vi>)
                      n226 = property on="ROI" class="Slide (strict)"("Scale.Visible"=FALSE) -> ()  [unwired: 2 in, 2 out]
                      n227 = Unbundle("ROI") -> (w391:dbl, w390:dbl)
                      n228 = property on="Property Node" class="Pict"(reference=w419) -> ("Height"=w400:u32, "Width"=w393:u32)  [unwired: 1 in, 2 out]
                      n229 = property on="Property Node" class="Pict"(reference=w419) -> ("Mouse"=w420:T8)  [unwired: 1 in, 2 out]
                      n230 = Unbundle By Name(w420) -> ("Mouse Position"=w401:cluster{"X":i32, "Y":i32})  [unwired: 1 out]
                      n231 = Bundle By Name(cluster=w401, "Y"=0, "X"=w384) -> (w407:cluster{"X":i32, "Y":i32})
                      n232 = Bundle By Name(cluster=w401, "Y"=w400, "X"=w384) -> (w402:cluster{"X":i32, "Y":i32})
                      n233 = Bundle By Name(cluster=w401, "Y"=0, "X"=w391) -> (w423:cluster{"X":i32, "Y":i32})
                      n234 = event shown="[1] \"ROI Scan\": Value Change" {
                        selector: _ -> [_ _]
                        dyn-events: _ -> [_ _]
                        timeout: 1 -> [_ _]
                        tunnel: w391 -> [_ w447]
                        tunnel: w390 -> [_ w446]
                        tunnel: [FALSE w438] -> w389
                        tunnel: [_ w436] -> w385
                        event Timeout {
                          n235 = event-data() -> ()  [unwired: 1 in, 3 out]
                        }
                        event "ROI Scan": Value Change {
                          n236 = event-data() -> ()  [unwired: 1 in, 6 out]
                          n237 = global read "configDB.vi" "scaleFactor"() -> (w434:dbl)
                          n238 = global read "configDB.vi" "slitPos"() -> (w435:i32)
                          n239 = Subtract(x=w447, y=w446) -> (x-y=w449:dbl)
                          n240 = Max & Min(x=w447, y=w446) -> (min(x,y)=w437:dbl)  [unwired: 1 out]
                          n241 = Absolute Value(x=w449) -> (abs(x)=w448:dbl)
                          n242 = Subtract(x=w437, y=w435) -> (x-y=w445:dbl)
                          n243 = Multiply(x=w448, y=w434) -> (x*y=w442:dbl)
                          n244 = Multiply(x=w445, y=w434) -> (x*y=w443:dbl)
                          n245 = Greater Or Equal To 0?(x=w443) -> (x >= 0?=w444:bool)
                          n246 = Divide(x=w442, y=sgl 1000.0) -> (x/y=w440:dbl)
                          n247 = case shown="True" w444 {
                            tunnel: w443 -> [w453 w461]
                            tunnel: [w451 w459] -> w439
                            tunnel: [w452 w460] -> w438
                            tunnel: [w450 w458] -> w436
                            frame False {
                              n248 = stacked-sequence {
                                tunnel: w453 -> [_ w456 _]
                                tunnel: [_ w455 _] -> w451
                                tunnel: [_ _ TRUE] -> w452
                                tunnel: [w454 _ _] -> w450
                                frame #0 {
                                n249 = call "queryStagePosition.vi"() -> ("stagePosition"=w454:string)  [unwired: 11 in]
                                }
                                frame #1 {
                                n250 = call "stageGoLeft.vi"("Step length (um)"=w456) -> ("Stage Position"=w455:string)  [unwired: 10 in]
                                }
                                frame #2 {
                                }
                              }
                            }
                            frame True {
                              n251 = stacked-sequence {
                                tunnel: w461 -> [_ w464 _]
                                tunnel: [_ w463 _] -> w459
                                tunnel: [_ _ TRUE] -> w460
                                tunnel: [w462 _ _] -> w458
                                frame #0 {
                                n252 = call "queryStagePosition.vi"() -> ("stagePosition"=w462:string)  [unwired: 11 in]
                                }
                                frame #1 {
                                n253 = call "stageGoRight.vi"("Step length (um)"=w464) -> ("Stage Position"=w463:string)  [unwired: 10 in]
                                }
                                frame #2 {
                                }
                              }
                            }
                          }
                          n254 = local write "Stage Position"(w439) -> ()
                          n255 = local write "Scan Length (mm)"(w440) -> ()
                        }
                      }
                      n256 = Bundle By Name(cluster=w401, "X"=w391, "Y"=w400) -> (w424:cluster{"X":i32, "Y":i32})
                      n257 = global read "configDB.vi" "leftCrop"() -> (w383:i32)
                      n258 = feedback #1() -> (w398:T9)  [unwired: 1 in]
                      n259 = disable-structure shown="Enabled" {
                        disable-tunnel: w432 -> [_ w496]
                        disable-tunnel: "ISO" -> [_ w495]
                        disable-tunnel: "Exposure Time" -> [_ w494]
                        disable-tunnel: [_ w491] -> w386
                        disable-tunnel: [_ w493] -> w409
                        disable-tunnel: w398 -> [_ w492]
                        frame Disabled {
                          n260 = Multiply(x="Exposure Time:", y=1) -> (x*y=→"ET Labelµ":dbl)
                          n261 = call "mightexLiveview.vi"("Blue Gain"="Blue Gain", "bright"="bright", "Green Gain"="Green Gain", "Red Gain"="Red Gain", "Gain?"="Gain?", "Exposure Time:"="Exposure Time:", "sharp"="sharp", "contrast"="contrast", "gamma"="gamma", "Close"=TRUE) -> ("new picture"=→"new picture":picture)  [unwired: 1 in]
                        }
                        frame Enabled {
                          n262 = property on="OM" class="Pict"() -> ("Draw Area Size"=w498:T10)  [unwired: 2 in, 2 out]
                          n263 = call "Empty Picture"() -> ("empty picture"=w490:picture)
                          n264 = call "canonLiveview.vi"("Shutter speed"=w494, "ISO"=w495, "inRef"=w496) -> ("output array"=w497:u32[][])  [unwired: 7 in, 1 out]
                          n265 = call <vilib>:"Flatten Pixmap.vi"("24-bit pixmap"=w497) -> ("image data"=w493:T9)  [unwired: 10 in]
                          n266 = Unbundle By Name(w492) -> ("Rectangle.bottom"=w501:i16, "Rectangle.right"=w499:i16)
                          n267 = Unbundle By Name(w498) -> ("Width"=w488:u32, "Height"=w500:u32)
                          n268 = Multiply(x=0.9, y=w488) -> (x*y=w485:dbl)
                          n269 = Subtract(x=w485, y=10.0) -> (x-y=w486:dbl)
                          n270 = property on="ROI" class="Slide (strict)"("Scale.Maximum"=w486, "Scale.Minimum"=10.0 ("Scale.Range:Minimum")) -> ()  [unwired: 2 in, 2 out]
                          n271 = call <vilib>:"Draw Flattened Pixmap.vi"("image data"=w492, "picture"=w490) -> ("new picture"=w491:picture)  [unwired: 7 in]
                          n272 = Divide(x=w488, y=w499) -> (x/y=w502:dbl)
                          n273 = Divide(x=w500, y=w501) -> (x/y=w503:dbl)
                          n274 = Max & Min(x=w502, y=w503) -> (min(x,y)=w504:dbl)  [unwired: 1 out]
                          n275 = property on="OM" class="Pict"("ZoomFactor"=w504) -> ()  [unwired: 2 in, 2 out]
                        }
                      }
                      n276 = call <vilib>:"Move Pen.vi"("new position"=w407, "picture"=w386) -> ("new picture"=w405:picture)  [unwired: 3 in]
                      n277 = call <vilib>:"Draw Line.vi"("picture"=w405, "end point"=w402, "color(black)"=w397, "pen"=T5 {"Width"=3, "Style"=enum."Dot"}) -> ("new picture"=w404:picture)  [unwired: 5 in]
                      n278 = call <vilib>:"Move Pen.vi"("new position"=w423, "picture"=w404) -> ("new picture"=w421:picture)  [unwired: 3 in]
                      n279 = Unbundle By Name(w409) -> ("Rectangle.left"=w418:i16, "Rectangle.top"=w417:i16, "Rectangle.right"=w416:i16, "Rectangle.bottom"=w415:i16, "Rectangle"=w413:T11)
                      n280 = global read "configDB.vi" "topCrop"() -> (w382:i32)
                      n281 = global read "configDB.vi" "rightCrop"() -> (w381:i32)
                      n282 = global read "configDB.vi" "bottomCrop"() -> (w380:i32)
                      n283 = call <vilib>:"Draw Line.vi"("picture"=w421, "end point"=w424, "color(black)"=w397, "pen"=w396) -> ("new picture"=w429:picture)  [unwired: 5 in]
                      n284 = Add(x=w417, y=w382) -> (x+y=w412:i32)
                      n285 = Subtract(x=w416, y=w381) -> (x-y=w411:i32)
                      n286 = Subtract(x=w415, y=w380) -> (x-y=w410:i32)
                      n287 = Add(x=w418, y=w383) -> (x+y=w414:i32)
                      n288 = global read "configDB.vi" "fovStart"() -> (w379:i32)
                      n289 = global read "configDB.vi" "fovEnd"() -> (w378:i32)
                      n290 = Bundle By Name(cluster=w413, "left"=w414, "top"=w412, "right"=w411, "bottom"=w410) -> (w408:T11)
                      n291 = call <vilib>:"Get Image Subset.vi"("subset rect"=w408, "image data"=w409) -> ("image subset"=w399:T9)  [unwired: 4 in, 1 out]
                      n292 = feedback-in #1(w399) -> ()
                      n293 = Bundle By Name(cluster=w401, "Y"=0, "X"=w390) -> (w426:cluster{"X":i32, "Y":i32})
                      n294 = Bundle By Name(cluster=w401, "Y"=w400, "X"=w390) -> (w428:cluster{"X":i32, "Y":i32})
                      n295 = call <vilib>:"Move Pen.vi"("new position"=w426, "picture"=w429) -> ("new picture"=w427:picture)  [unwired: 3 in]
                      n296 = call <vilib>:"Draw Line.vi"("picture"=w427, "end point"=w428, "color(black)"=w397, "pen"=w396) -> ("new picture"=w394:picture)  [unwired: 5 in]
                      n297 = call "drawHorizontalRange.vi"("Y 2"=w378, "Y"=w379, "Xmax"=w393, "picture"=w394) -> ("new picture"=→"OM":picture)  [unwired: 7 in]
                    }
                  }
                  n298 = case shown="True" w282 {
                    tunnel: [FALSE w291] -> w289
                    frame False {
                    }
                    frame True {
                      n299 = call <userlib>:"GetStatus.vi"() -> ("status"=w295:T2)  [unwired: 3 in, 2 out]
                      n300 = local read "Live View"() -> (w292:bool)
                      n301 = Equal?(x=w295, y=Error_Code_Enum_typedef."DRV_IDLE" ("status")) -> (x = y?=w293:bool)
                      n302 = And(x=w293, y=w292) -> (x .and. y?=w291:bool)
                    }
                  }
                  n303 = case shown="True" w289 {
                    frame False {
                    }
                    frame True {
                      n304 = flat-sequence {
                        frame #0 {
                          n305 = call "ixonLiveview.vi"("stop"=TRUE) -> ("Left Graph"=→"Left Graph":i32[][])  [unwired: 10 in]
                        }
                        frame #1 {
                          n306 = local read "left Coords"() -> (w302:T1)
                          n307 = local read "Line Profile"() -> (w304:string)
                          n308 = local read "line avg?"() -> (w303:bool)
                          n309 = control-ref of="Left Graph"() -> (w305:refnum<vi>)
                          n310 = property on="Property Node" class="IntGraph (strict)"(reference=w305) -> ("Value"=w300:i32[][])  [unwired: 1 in, 2 out]
                          n311 = local read "left color 2"() -> (w299:u32)
                          n312 = case shown="\"Horizontal\", Default" w304 {
                            tunnel: w300 -> [w313 w341]
                            tunnel: [w312 w346] -> w301
                            tunnel: w303 -> [w314 w345]
                            tunnel: w305 -> [w309 w343]
                            tunnel: w304 -> [w311 w344]
                            tunnel: w302 -> [w310 w342]
                            tunnel: w299 -> [w308 w340]
                            tunnel: [w307 w339] -> w298
                            frame "Vertical" {
                              n313 = case shown="False" w314 {
                                tunnel: w313 -> [w324 w331]
                                tunnel: [w323 w329] -> w312
                                tunnel: w309 -> [w315 w328]
                                tunnel: w311 -> [w325 _]
                                tunnel: w310 -> [w322 _]
                                tunnel: w308 -> [w321 _]
                                tunnel: [w316 0] -> w307
                                frame False {
                                n314 = property class="IntGraph (strict)"(reference=w315) -> ("XScale.Multiplier"=w319:dbl, "XScale.Offset"=w317:dbl)  [unwired: 1 in, 2 out]
                                n315 = call "drawIntensityGraph.vi"("color(black)"=w321, "Combo Box"=w325, "Coords"=w322, "Left Graph 2"=w315) -> ("x"=w320:i32)  [unwired: 6 in, 1 out]
                                n316 = Index Array(array=w324, index (col)=w320) -> (element=w323:i32[])  [unwired: 1 in]
                                n317 = Multiply(x=w320, y=w319) -> (x*y=w318:dbl)
                                n318 = Add(x=w318, y=w317) -> (x+y=w316:dbl)
                                }
                                frame True {
                                n319 = call "Empty Picture"() -> ("empty picture"=w327:picture)
                                n320 = for {
                                N: 512 -> [_]
                                tunnel: w331 -> [w337]
                                tunnel: [w333] -> w329 mode=indexing
                                i -> [w332]
                                n321 = Index Array(array=w337, index (row)=w332) -> (element=w336:i32[])  [unwired: 1 in]
                                n322 = Add Array Elements(numeric array=w336) -> (sum=w335:i32)
                                n323 = Divide(x=w335, y=384) -> (x/y=w333:dbl)
                                }
                                n324 = property on="Property Node" class="IntGraph (strict)"(reference=w328, "PlotImages.Front"=w327) -> ()  [unwired: 1 in, 2 out]
                                }
                              }
                              n325 = property on="left profie location" class="DigNum (strict)"("Caption.Text"="Wavelength" ("Label.Text")) -> ()  [unwired: 2 in, 2 out]
                            }
                            frame "Horizontal", Default {
                              n326 = case shown="False" w345 {
                                tunnel: w341 -> [w356 w362]
                                tunnel: [w355 w361] -> w346
                                tunnel: w344 -> [w357 _]
                                tunnel: w343 -> [w352 w359]
                                tunnel: w342 -> [w354 _]
                                tunnel: w340 -> [w353 _]
                                tunnel: [w347 0] -> w339
                                frame False {
                                n327 = property class="IntGraph (strict)"(reference=w352) -> ("YScale.Multiplier"=w351:dbl, "YScale.Offset"=w349:dbl)  [unwired: 1 in, 2 out]
                                n328 = call "drawIntensityGraph.vi"("color(black)"=w353, "Combo Box"=w357, "Coords"=w354, "Left Graph 2"=w352) -> ("y"=w348:i32)  [unwired: 6 in, 1 out]
                                n329 = Index Array(array=w356, index (row)=w348) -> (element=w355:i32[])  [unwired: 1 in]
                                n330 = Multiply(x=w348, y=w351) -> (x*y=w350:dbl)
                                n331 = Add(x=w350, y=w349) -> (x+y=w347:dbl)
                                }
                                frame True {
                                n332 = call "Empty Picture"() -> ("empty picture"=w360:picture)
                                n333 = for {
                                N: 384 -> [_]
                                tunnel: w362 -> [w369]
                                tunnel: [w364] -> w361 mode=indexing
                                i -> [w368]
                                n334 = Index Array(array=w369, index (col)=w368) -> (element=w367:i32[])  [unwired: 1 in]
                                n335 = Add Array Elements(numeric array=w367) -> (sum=w366:i32)
                                n336 = Divide(x=w366, y=512) -> (x/y=w364:dbl)
                                }
                                n337 = property on="Property Node" class="IntGraph (strict)"(reference=w359, "PlotImages.Front"=w360) -> ()  [unwired: 1 in, 2 out]
                                }
                              }
                              n338 = property on="left profie location" class="DigNum (strict)"("Caption.Text"="Y" ("Label.Text")) -> ()  [unwired: 2 in, 2 out]
                            }
                          }
                          n339 = local write "left profie location"(w298) -> ()
                          n340 = local write "left wvf graph"(w301) -> ()
                        }
                      }
                    }
                  }
                }
                frame #2 {
                  n341 = control-ref of="left wvf graph"() -> (w515:refnum<vi>)
                  n342 = control-ref of="right wvf graph"() -> (w512:refnum<vi>)
                  n343 = call "waveformGraphDraw.vi"("color(black)"="left wvf color 3", "WaveMouse 2"="left WaveMouse", "right wvf graph 2"=w515) -> ("Wavelength 2"=w506:dbl, "Intensity 2"=→"Intensity":i32)  [unwired: 7 in]
                  n344 = call "waveformGraphDraw.vi"("color(black)"="right wvf color 4", "WaveMouse 2"="right WaveMouse 2", "right wvf graph 2"=w512) -> ("Wavelength 2"=w505:dbl, "Intensity 2"=→"Intensity 2":i32)  [unwired: 7 in]
                  n345 = local write "left Wavelength"(w506) -> ()
                  n346 = local write "right Wavelength"(w505) -> ()
                  n347 = global read "applicationControl.vi" "hasIxon"() -> (w507:bool)
                  n348 = case shown="True" w507 {
                    frame False {
                    }
                    frame True {
                      n349 = call <userlib>:"GetTemperature.vi"() -> ("status"=w518:T2, "temperature"=w519:i32)  [unwired: 4 in, 2 out]
                      n350 = Equal?(x=w518, y=Error_Code_Enum_typedef."DRV_TEMPERATURE_STABILIZED") -> (x = y?=w516:bool)
                      n351 = case shown="True" w516 {
                        frame False {
                          n352 = local write "Cooler"(FALSE ("Cooler")) -> ()
                        }
                        frame True {
                          n353 = local write "Cooler"(TRUE ("Cooler")) -> ()
                        }
                      }
                      n354 = local write "Temperature"(w519) -> ()
                      n355 = local write "temp. status 2"(w518) -> ()
                    }
                  }
                }
              }
              n356 = local read "Read mode"() -> (w214:bool)
              n357 = local read "Shut Down"() -> (w221:bool)
              n358 = Or(x="Scan Start", y=w221) -> (x .or. y?=w219:bool)
              n359 = Or(x=w219, y=w218) -> (x .or. y?=w216:bool)
              n360 = Or(x=w214, y=w216) -> (x .or. y?=w215:bool)
            }
          }
          frame #2 {
            w533 = FALSE ("Visible")
            w526 = TRUE ("Visible")
            w537 = T4."Disabled and Grayed Out" ("Disabled")
            n361 = property on="Right Graph" class="IntGraph (strict)"("Caption.Text"="Object Image") -> ()  [unwired: 2 in, 2 out]
            n362 = invoke on="Right Graph" class="IntGraph (strict)" method="Reinit To Default"() -> ()  [unwired: 3 in, 3 out]
            n363 = local write "Right Graph"(i32[][] [] ("Right Graph")) -> ()
            n364 = property on="Go back after scan" class="Bool (strict)"("DisabledEnum"=w537) -> ()  [unwired: 2 in, 2 out]
            n365 = property on="Shutter Control" class="Enum (strict)"("DisabledEnum"=w537) -> ()  [unwired: 2 in, 2 out]
            n366 = property on="go left Button" class="Bool"("DisabledEnum"=w537) -> ()  [unwired: 2 in, 2 out]
            n367 = property on="HSS (MHz)" class="Ring (strict)"("DisabledEnum"=w537) -> ()  [unwired: 2 in, 2 out]
            n368 = property on="VSS (s)" class="Ring (strict)"("DisabledEnum"=w537) -> ()  [unwired: 2 in, 2 out]
            n369 = property on="Live View" class="Bool (strict)"("DisabledEnum"=w537) -> ()  [unwired: 2 in, 2 out]
            n370 = call "queryStagePosition.vi"() -> ("stagePosition"=w535:string)  [unwired: 11 in]
            n371 = property on="Current \nScan Frame" class="DigNum (strict)"("Visible"=w526) -> ()  [unwired: 2 in, 2 out]
            n372 = property on="Scan Abort" class="Bool (strict)"("DisabledEnum"=T4."Enabled" ("Disabled")) -> ()  [unwired: 2 in, 2 out]
            n373 = property on="Total \nScan Frame" class="DigNum (strict)"("Visible"=w526) -> ()  [unwired: 2 in, 2 out]
            n374 = property on="Exposure Time (s)" class="DigNum (strict)"("DisabledEnum"=w537) -> ()  [unwired: 2 in, 2 out]
            n375 = property on="Step length (um)" class="DigNum (strict)"("DisabledEnum"=w537) -> ()  [unwired: 2 in, 2 out]
            n376 = property on="Take shot" class="Bool (strict)"("DisabledEnum"=w537) -> ()  [unwired: 2 in, 2 out]
            n377 = property on="Scan Length (mm)" class="DigNum (strict)"("DisabledEnum"=w537) -> ()  [unwired: 2 in, 2 out]
            n378 = property on="Scan Start" class="Bool"("DisabledEnum"=w537) -> ()  [unwired: 2 in, 2 out]
            n379 = property on="go right Button" class="Bool"("DisabledEnum"=w537) -> ()  [unwired: 2 in, 2 out]
            n380 = property on="Scan Step (um)" class="DigNum (strict)"("DisabledEnum"=w537) -> ()  [unwired: 2 in, 2 out]
            n381 = property on="Right Graph" class="IntGraph (strict)"("Visible"=w526) -> ()  [unwired: 2 in, 2 out]
            n382 = local write "left wvf graph"(i32[] [] ("Waveform Graph")) -> ()
            n383 = local read "Shut Down"() -> (w524:bool)
            n384 = local read "Read mode"() -> (w523:bool)
            n385 = global read "applicationControl.vi" "hasCanon"() -> (w525:bool)
            n386 = flat-sequence {
              tunnel: w534 -> [w541]
              tunnel: w525 -> [w540]
              frame #0 {
                n387 = case shown="True" w540 {
                  tunnel: w541 -> [_ w542]
                  frame False {
                  }
                  frame True {
                    n388 = call "closeCanon.vi"("inCameraRef"=w542) -> ()  [unwired: 11 in]
                  }
                }
              }
              frame #1 {
                n389 = disable-structure shown="Enabled" {
                  frame Disabled {
                    n390 = property on="Right Graph" class="IntGraph (strict)"("XScale.ScaleFit"=u8 0 ("X Scale.Scale Fit")) -> ()  [unwired: 2 in, 2 out]
                  }
                  frame Enabled {
                  }
                }
                n391 = Wait (ms)(milliseconds to wait=u32 250) -> ()  [unwired: 1 out]
              }
              frame #2 {
                n392 = local read "Scan Step (um)"() -> (w546:dbl)
                n393 = property on="Scan Length (mm)" class="DigNum (strict)"() -> ("Value"=w552:dbl)  [unwired: 2 in, 2 out]
                n394 = Divide(x=w546, y=1000.0) -> (x/y=w547:dbl)
                n395 = property on="Right Graph" class="IntGraph (strict)"("XScale.Offset"=0.0 ("X Scale.Offset and Multiplier:Offset"), "XScale.Multiplier"=w547, "XScale.NameLbl.Text"="X (mm)" ("X Scale.Name Label.Text")) -> (error out=w545:errorcluster)  [unwired: 2 in, 1 out]
                n396 = property on="Right Graph" class="IntGraph (strict)"(error in=w545, "XScale.Maximum"=w552, "XScale.Minimum"=0.0 ("X Scale.Range:Minimum")) -> ()  [unwired: 1 in, 2 out]
              }
              frame #3 {
                n397 = disable-structure shown="Enabled" {
                  frame Enabled {
                    n398 = property on="Right Graph" class="IntGraph (strict)"("XScale.ScaleFit"=u8 0 ("X Scale.Scale Fit")) -> ()  [unwired: 2 in, 2 out]
                  }
                  frame Disabled {
                  }
                }
              }
            }
            n399 = Or(x=w524, y=w523) -> (x .or. y?=w522:bool)
            n400 = case shown="True" w522 {
              frame False {
              }
              frame True {
                n401 = local write "Scan Length (mm)"(0.0 ("Scan Length (mm)")) -> ()
              }
            }
            n402 = control-ref of="ROI Scan"() -> (w531:refnum<vi>)
            n403 = control-ref of="Exposure Time"() -> (w530:refnum<vi>)
            n404 = property on="Property Node" class="Ring (strict)"(reference=w530, "Visible"=w533) -> ()  [unwired: 1 in, 2 out]
            n405 = property on="Property Node" class="Bool"(reference=w531, "Visible"=w533) -> ()  [unwired: 1 in, 2 out]
            n406 = control-ref of="ROI"() -> (w532:refnum<vi>)
            n407 = control-ref of="OM"() -> (w528:refnum<vi>)
            n408 = property on="Property Node" class="Slide (strict)"(reference=w532, "Visible"=w533) -> ()  [unwired: 1 in, 2 out]
            n409 = control-ref of="ISO"() -> (w529:refnum<vi>)
            n410 = property on="Property Node" class="Pict"(reference=w528, "Visible"=w533) -> ()  [unwired: 1 in, 2 out]
            n411 = property on="Property Node" class="Ring (strict)"(reference=w529, "Visible"=w533) -> ()  [unwired: 1 in, 2 out]
          }
          frame #3 {
            n412 = local read "Scan Length (mm)"() -> (w556:dbl)
            n413 = while {
              stop <- w575 stop-if-true
              n414 = disable-structure shown="Disabled" {
                frame Disabled {
                  n415 = global read "displayImage.vi" "On Sensor Image"() -> (w578:i32[][])
                  n416 = local write "Left Graph"(w578) -> ()
                }
                frame Enabled {
                }
              }
              n417 = disable-structure shown="Disabled" {
                frame Disabled {
                  n418 = global read "applicationControl.vi" "currentScanFrame"() -> (w577:dbl)
                  n419 = global read "applicationControl.vi" "totalScanFrame"() -> (w576:dbl)
                  n420 = local write "Current \nScan Frame"(w577) -> ()
                  n421 = local write "Total \nScan Frame"(w576) -> ()
                }
                frame Enabled {
                }
              }
              n422 = local read "Scanning done"() -> (w575:bool)
            }
            n423 = local read "Scan Step (um)"() -> (w555:dbl)
            n424 = global write "imageSettings.vi" "realXDimension"(w556) -> ()
            n425 = global write "imageSettings.vi" "stepLength"(w555) -> ()
            n426 = flat-sequence {
              tunnel: w556 -> [w583]
              tunnel: w555 -> [w584]
              tunnel: "Go back after scan" -> [w585]
              tunnel: [w585] -> w571
              tunnel: [w584] -> w570
              tunnel: [w583] -> w569
              tunnel: [w579] -> w568
              tunnel: w564 -> [w591]
              tunnel: w571 -> [w590]
              tunnel: w570 -> [w589]
              tunnel: w569 -> [w588]
              tunnel: w568 -> [w587]
              tunnel: w561 -> [w586]
              tunnel: w562 -> [w598]
              frame #0 {
                n427 = Open VI Reference(vi path="ixonScan.vi") -> (vi reference=w582:refnum<vi>)  [unwired: 5 in, 1 out]
                n428 = invoke class="VI" method="Default Vals.Reinit All"(reference=w582) -> (reference out=w581:refnum<vi>)  [unwired: 2 in, 2 out]
                n429 = local read "Shut Down"() -> (w579:bool)
                n430 = Close Reference(reference=w581) -> ()  [unwired: 1 in, 1 out]
              }
              frame #1 {
                n431 = case shown="False" w587 {
                  tunnel: w591 -> [w597 _]
                  tunnel: w590 -> [w596 _]
                  tunnel: w589 -> [w595 _]
                  tunnel: w588 -> [w594 _]
                  tunnel: w586 -> [w593 _]
                  frame False {
                    n432 = call "ixonScan.vi"("output cluster"=w593, "stageReturnPosition"=w597, "goBackAfterScan"=w596, "scanStep"=w595, "scanLength"=w594) -> ()  [unwired: 4 in, 3 out]
                    "scanned?" <- TRUE ("Scanned?")
                  }
                  frame True {
                  }
                }
              }
              frame #2 {
                w599 = FALSE ("Scan Abort")
                n433 = local write "Scanning done"(TRUE) -> ()
                n434 = local write "Scan Abort"(w599) -> ()
                n435 = global write "applicationControl.vi" "scanAbort"(w599) -> ()
                n436 = property class="Slide (strict)"(reference=w598, "Visible"=w599) -> ()  [unwired: 1 in, 2 out]
              }
            }
            n437 = control-ref of="Scan Abort"() -> (w563:refnum<vi>)
            n438 = control-ref of="Constructing data"() -> (w562:refnum<vi>)
            n439 = control-ref of="Current \nScan Frame"() -> (w557:refnum<vi>)
            n440 = control-ref of="Total \nScan Frame"() -> (w558:refnum<vi>)
            n441 = control-ref of="Left Graph"() -> (w559:refnum<vi>)
            n442 = control-ref of="Right Graph"() -> (w560:refnum<vi>)
            n443 = case shown="True" w567 {
              tunnel: w566 -> [_ w574]
              tunnel: w565 -> [w573 _]
              tunnel: [w573 w574] -> w564
              frame False {
              }
              frame True {
              }
            }
            n444 = Bundle("Scan Abort"=w563, "Constructing data"=w562, "Right Graph"=w560, "Left Graph"=w559, "Total \nScan Frame"=w558, "Current \nScan Frame"=w557) -> (w561:T12)  [unwired: 1 in]
          }
          frame #4 {
            n445 = flat-sequence {
              tunnel: [w613] -> w601
              tunnel: [w625] -> w602
              tunnel: w601 -> [w624]
              tunnel: [w1107] -> w603
              tunnel: w602 -> [w1107]
              frame #0 {
                w607 = TRUE ("Visible")
                w608 = FALSE ("Visible")
                w605 = T4."Disabled and Grayed Out" ("Disabled")
                w604 = T4."Enabled" ("Disabled")
                n446 = global read "applicationControl.vi" "hasIxon"() -> (w606:bool)
                n447 = global read "imageSettings.vi" "specArray"() -> (w612:sgl[])
                n448 = invoke on="Y" class="DigNum (strict)" method="Reinit To Default"() -> ()  [unwired: 3 in, 3 out]
                n449 = invoke on="X" class="DigNum (strict)" method="Reinit To Default"() -> ()  [unwired: 3 in, 3 out]
                n450 = case shown="False" w606 {
                  tunnel: w605 -> [w619 _]
                  frame False {
                    n451 = property on="Wipe and Quit" class="Bool"("DisabledEnum"=w619) -> ()  [unwired: 2 in, 2 out]
                  }
                  frame True {
                  }
                }
                n452 = property on="Set Origin" class="Bool"("DisabledEnum"=w605) -> ()  [unwired: 2 in, 2 out]
                n453 = property on="right wvf graph" class="WFGraph (strict)"("Caption.Text"="Point Spectra") -> ()  [unwired: 2 in, 2 out]
                n454 = property on="Go Origin" class="Bool"("DisabledEnum"=w605) -> ()  [unwired: 2 in, 2 out]
                n455 = Array Max & Min(array=w612) -> (max value=w611:sgl, min value=w610:sgl)  [unwired: 2 out]
                n456 = property on="Wavelength slide" class="Slide (strict)"("Scale.Maximum"=w611, "Scale.Minimum"=w610) -> ()  [unwired: 2 in, 2 out]
                n457 = invoke on="Left Graph" class="IntGraph (strict)" method="Reinit To Default"() -> ()  [unwired: 3 in, 3 out]
                n458 = property on="Right Graph" class="IntGraph (strict)"("XScale.ScaleFit"=u8 2 ("X Scale.Scale Fit")) -> ()  [unwired: 2 in, 2 out]
                n459 = property on="Substract Background" class="Bool (strict)"("Visible"=w607) -> ()  [unwired: 2 in, 2 out]
                n460 = property on="Background" class="Bool"("DisabledEnum"=w605) -> ()  [unwired: 2 in, 2 out]
                n461 = property on="Y" class="DigNum (strict)"("Visible"=w607) -> ()  [unwired: 2 in, 2 out]
                n462 = property on="Divide Reference" class="Bool (strict)"("Visible"=w607) -> ()  [unwired: 2 in, 2 out]
                n463 = property on="X" class="DigNum (strict)"("Visible"=w607) -> ()  [unwired: 2 in, 2 out]
                n464 = property on="Total \nScan Frame" class="DigNum (strict)"("Visible"=w608) -> ()  [unwired: 2 in, 2 out]
                n465 = property on="Current \nScan Frame" class="DigNum (strict)"("Visible"=w608) -> ()  [unwired: 2 in, 2 out]
                n466 = property on="Bandwidth (Frame)" class="DigNum (strict)"("DisabledEnum"=w604) -> ()  [unwired: 2 in, 2 out]
                n467 = property on="Path" class="Path"("DisabledEnum"=w604) -> ()  [unwired: 2 in, 2 out]
                n468 = property on="left wvf graph" class="WFGraph (strict)"("DisabledEnum"=w604) -> ()  [unwired: 2 in, 2 out]
                n469 = property on="Wipe and Quit" class="Bool"("DisabledEnum"=w604) -> ()  [unwired: 2 in, 2 out]
                n470 = property on="Save File" class="Bool (strict)"("DisabledEnum"=w604) -> ()  [unwired: 2 in, 2 out]
                n471 = property on="Wavelength slide" class="Slide (strict)"("DisabledEnum"=w604) -> ()  [unwired: 2 in, 2 out]
                n472 = global read "imageSettings.vi" "backgroundExist"() -> (w613:bool)
                n473 = case shown="True" w613 {
                  tunnel: [T4."Disabled and Grayed Out" ("Disabled") T4."Enabled" ("Disabled")] -> w616
                  frame False {
                  }
                  frame True {
                  }
                }
                n474 = global read "imageSettings.vi" "referenceExist"() -> (w614:bool)
                n475 = case shown="False" w614 {
                  tunnel: [T4."Disabled and Grayed Out" ("Disabled") T4."Enabled" ("Disabled")] -> w615
                  frame False {
                  }
                  frame True {
                  }
                }
                n476 = property on="Substract Background" class="Bool (strict)"("DisabledEnum"=w616) -> ()  [unwired: 2 in, 2 out]
                n477 = property on="graph real ratio?" class="Bool (strict)"("Visible"=w607) -> ()  [unwired: 2 in, 2 out]
                n478 = property on="Divide Reference" class="Bool (strict)"("DisabledEnum"=w615) -> ()  [unwired: 2 in, 2 out]
                n479 = property on="Wavelength slide" class="Slide (strict)"("Visible"=w607) -> ()  [unwired: 2 in, 2 out]
                n480 = local write "Scanning done"(FALSE ("Scanning done")) -> ()
                n481 = property on="Bandwidth (Frame)" class="DigNum (strict)"("Visible"=w607) -> ()  [unwired: 2 in, 2 out]
                n482 = property on="Set Temperature" class="DigNum (strict)"("DisabledEnum"=w605) -> ()  [unwired: 2 in, 2 out]
                n483 = property on="Read mode" class="Bool (strict)"("DisabledEnum"=w605) -> ()  [unwired: 2 in, 2 out]
                n484 = property on="Read File" class="Bool (strict)"("DisabledEnum"=w604) -> ()  [unwired: 2 in, 2 out]
                n485 = property on="OM" class="Bool (strict)"("DisabledEnum"=w605) -> ()  [unwired: 2 in, 2 out]
                n486 = property on="Scan Abort" class="Bool (strict)"("DisabledEnum"=w605) -> ()  [unwired: 2 in, 2 out]
                n487 = property on="Reference" class="Bool"("DisabledEnum"=w605) -> ()  [unwired: 2 in, 2 out]
              }
              frame #1 {
                n488 = in-place {
                  in-place-border: [w628] -> w625
                  in-place-border: [w627] -> _
                  in-place-border: w624 -> [w626]
                  n489 = while {
                    tunnel: [w642] -> w628
                    tunnel: [w643] -> w627
                    tunnel: w626 -> [w662]
                    stop <- w669 stop-if-true
                    # "wavelength"
                    n490 = global read "configDB.vi" "specMultiplier"() -> (w655:dbl)
                    n491 = global read "configDB.vi" "specOffset"() -> (w656:dbl)
                    n492 = global read "configDB.vi" "xPixels"() -> (w637:i32)
                    n493 = case shown="False" "Divide Reference" {
                      tunnel: [w750 w758] -> w665
                      tunnel: "Substract Background" -> [w749 _]
                      tunnel: w662 -> [w748 _]
                      frame False {
                        n494 = case shown="False" w749 {
                          tunnel: [w752 w754] -> w750
                          frame False {
                            n495 = call "dataCube.vi"("Enum"=enum16{"clear", "read", "write"}."read") -> ("imageCubeOut"=w752:i32[][][])  [unwired: 8 in, 2 out]
                          }
                          frame True {
                            n496 = call "dataCube.vi"("Enum"=enum16{"clear", "read", "write"}."read") -> ("imageCubeBkgSubstracted"=w754:i32[][][])  [unwired: 8 in, 2 out]
                          }
                        }
                        n497 = case shown="True" w748 {
                          frame False {
                          }
                          frame True {
                            n498 = property on="Substract Background" class="Bool (strict)"("DisabledEnum"=T4."Enabled" ("Disabled")) -> ()  [unwired: 2 in, 2 out]
                          }
                        }
                      }
                      frame True {
                        n499 = call "dataCube.vi"("Enum"=enum16{"clear", "read", "write"}."read") -> ("imageCubeBkgSubstractedRefDivided"=w758:i32[][][])  [unwired: 8 in, 2 out]
                        n500 = property on="Substract Background" class="Bool (strict)"("Value"=TRUE ("Substract Background"), "DisabledEnum"=T4."Disabled and Grayed Out" ("Disabled")) -> ()  [unwired: 2 in, 2 out]
                      }
                    }
                    n501 = event shown="[8] Timeout" {
                      selector: _ -> [_ _ _ _ _ _ _ _ _]
                      dyn-events: _ -> [_ _ _ _ _ _ _ _ _]
                      timeout: 10 -> [_ _ _ _ _ _ _ _ _]
                      tunnel: w665 -> [w825 w896 w969 _ _ _ _ _ _]
                      tunnel: [w812 w883 w956 _ _ _ _ _ w1098] -> w631
                      tunnel: [w811 w882 w955 _ _ _ _ _ w1097] -> w630
                      tunnel: [w793 w864 w937 w990 w1010 FALSE w1035 w1092 w1096] -> w642
                      tunnel: [w793 w864 w937 w990 FALSE w1023 w1035 w1092 w1096] -> w643
                      event "Right Graph": Mouse Down {
                        w793 = FALSE
                        # "<-- asymmetry"
                        # "Needed because panel (0,0) is at TOP left rather than bottom left."
                        n502 = event-data() -> ("Coords"=w791:T1)  [unwired: 1 in]
                        n503 = call "Empty Picture"() -> ("empty picture"=w802:picture)
                        n504 = local write "right Coords"(w791) -> ()
                        n505 = control-ref of="Right Graph"() -> (w804:refnum<vi>)
                        n506 = property on="Property Node" class="IntensityGraph (strict)"(reference=w804, "PlotImages.Front"=w802) -> ("Height"=w806:u32, "PlotImages.Front"=w800:picture)  [unwired: 1 in, 2 out]
                        n507 = property on="Property Node" class="IntensityGraph (strict)"(reference=w804) -> ("X Scale.Range:Maximum"=w829:dbl, "X Scale.Range:Minimum"=w828:dbl, "Plot Area:Size:Width"=w827:u32, "Plot Area:Position:Left"=w826:i32)  [unwired: 1 in, 2 out]
                        n508 = property on="Property Node" class="IntensityGraph (strict)"(reference=w804) -> ("Y Scale.Range:Maximum"=w851:dbl, "Y Scale.Range:Minimum"=w846:dbl, "Plot Area:Size:Height"=w845:u32, "Plot Area:Position:Top"=w838:i32)  [unwired: 1 in, 2 out]
                        n509 = Unbundle By Name(w791) -> ("Horizontal"=w807:i32)
                        n510 = Unbundle By Name(w791) -> ("Vertical"=w850:i32)
                        n511 = To Double Precision Float(number=w850) -> (double precision float=w844:dbl)
                        n512 = To Double Precision Float(number=w807) -> (double precision float=w833:dbl)
                        n513 = To Double Precision Float(number=w826) -> (double precision float=w834:dbl)
                        n514 = To Double Precision Float(number=w838) -> (double precision float=w843:dbl)
                        n515 = To Double Precision Float(number=w827) -> (double precision float=w837:dbl)
                        n516 = To Double Precision Float(number=w845) -> (double precision float=w839:dbl)
                        n517 = Subtract(x=w833, y=w834) -> (x-y=w797:dbl)
                        n518 = Bundle By Name(cluster=w791, "Horizontal"=w797, "Vertical"=0) -> (w808:T1)
                        n519 = Bundle By Name(cluster=w791, "Horizontal"=w797, "Vertical"=w806) -> (w805:T1)
                        n520 = Subtract(x=w844, y=w843) -> (x-y=w796:dbl)
                        n521 = Bundle By Name(cluster=w791, "Horizontal"=w797, "Vertical"=w796) -> (w798:T1)
                        n522 = call <vilib>:"Draw Point.vi"("picture"=w800, "point(x,y)"=w798, "color(black)"="right color", "pen"=T5 {"Width"=6, "Style"=enum."Solid"}) -> ("new picture"=w799:picture)  [unwired: 5 in]
                        n523 = call <vilib>:"Move Pen.vi"("new position"=w808, "picture"=w799) -> ("new picture"=w810:picture)  [unwired: 3 in]
                        n524 = Subtract(x=w839, y=w796) -> (x-y=w842:dbl)
                        n525 = In Range and Coerce(upper limit=w837, x=w797, lower limit=0.0) -> (coerced(x)=w836:dbl)  [unwired: 1 out]
                        n526 = In Range and Coerce(upper limit=w839, x=w842, lower limit=0.0) -> (coerced(x)=w840:dbl)  [unwired: 1 out]
                        n527 = call <vilib>:"Draw Line.vi"("picture"=w810, "end point"=w805, "color(black)"="right color", "pen"=T5 {"Width"=2, "Style"=enum."Dash"}) -> ("new picture"=w803:picture)  [unwired: 5 in]
                        n528 = Subtract(x=w829, y=w828) -> (x-y=w830:dbl)
                        n529 = Divide(x=w836, y=w837) -> (x/y=w831:dbl)
                        n530 = Subtract(x=w851, y=w846) -> (x-y=w849:dbl)
                        n531 = Divide(x=w840, y=w839) -> (x/y=w848:dbl)
                        n532 = Multiply(x=w830, y=w831) -> (x*y=w832:dbl)
                        n533 = Multiply(x=w849, y=w848) -> (x*y=w847:dbl)
                        n534 = property on="Property Node" class="IntensityGraph (strict)"(reference=w804, "PlotImages.Front"=w803) -> ()  [unwired: 1 in, 2 out]
                        n535 = property on="Right Graph" class="IntGraph (strict)"() -> ("XScale.Multiplier"=w820:dbl, "XScale.Offset"=w822:dbl, "YScale.Multiplier"=w815:dbl, "YScale.Offset"=w817:dbl)  [unwired: 2 in, 2 out]
                        n536 = Add(x=w832, y=w828) -> (x+y=w812:dbl)
                        n537 = Add(x=w847, y=w846) -> (x+y=w811:dbl)
                        n538 = Subtract(x=w811, y=w817) -> (x-y=w816:dbl)
                        n539 = Subtract(x=w812, y=w822) -> (x-y=w821:dbl)
                        n540 = Divide(x=w816, y=w815) -> (x/y=w814:dbl)
                        n541 = Divide(x=w821, y=w820) -> (x/y=w819:dbl)
                        n542 = Round To Nearest(number=w814) -> (nearest integer value=w813:dbl)
                        n543 = Round To Nearest(number=w819) -> (nearest integer value=w818:dbl)
                        n544 = Index Array(array=w825, index (dim 1)=w813, index (dim 2)=w818) -> (element=w794:i32[])  [unwired: 1 in]
                        n545 = local write "right wvf graph"(w794) -> ()
                        n546 = Index Array(array=w825, index (dim 2)=w818) -> (element=w824:i32[][])  [unwired: 2 in]
                        n547 = Transpose 2D Array(2D array=w824) -> (transposed array=w823:i32[][])
                        n548 = local write "Left Graph"(w823) -> ()
                      }
                      event "X": Value Change {
                        w864 = FALSE
                        # "<-- asymmetry"
                        # "Needed because panel (0,0) is at TOP left rather than bottom left."
                        n549 = event-data() -> ("NewVal"=w862:dbl)  [unwired: 1 in]
                        n550 = local read "right Coords"() -> (w863:T1)
                        n551 = local read "right color"() -> (w853:u32)
                        n552 = control-ref of="Right Graph"() -> (w875:refnum<vi>)
                        n553 = property on="Property Node" class="IntensityGraph (strict)"(reference=w875) -> ("X Scale.Range:Maximum"=w900:dbl, "X Scale.Range:Minimum"=w899:dbl, "Plot Area:Size:Width"=w898:u32, "Plot Area:Position:Left"=w897:i32)  [unwired: 1 in, 2 out]
                        n554 = property on="Property Node" class="IntensityGraph (strict)"(reference=w875) -> ("Y Scale.Range:Maximum"=w919:dbl, "Y Scale.Range:Minimum"=w914:dbl, "Plot Area:Size:Height"=w913:u32, "Plot Area:Position:Top"=w906:i32)  [unwired: 1 in, 2 out]
                        n555 = call "Empty Picture"() -> ("empty picture"=w873:picture)
                        n556 = property on="Property Node" class="IntensityGraph (strict)"(reference=w875, "PlotImages.Front"=w873) -> ("Height"=w877:u32, "PlotImages.Front"=w871:picture)  [unwired: 1 in, 2 out]
                        n557 = To Double Precision Float(number=w897) -> (double precision float=w857:dbl)
                        n558 = To Double Precision Float(number=w906) -> (double precision float=w911:dbl)
                        n559 = To Double Precision Float(number=w898) -> (double precision float=w859:dbl)
                        n560 = To Double Precision Float(number=w913) -> (double precision float=w907:dbl)
                        n561 = Subtract(x=w900, y=w899) -> (x-y=w861:dbl)
                        n562 = Divide(x=w862, y=w861) -> (x/y=w860:dbl)
                        n563 = Multiply(x=w860, y=w859) -> (x*y=w858:dbl)
                        n564 = Add(x=w858, y=w857) -> (x+y=w856:dbl)
                        n565 = Round To Nearest(number=w856) -> (nearest integer value=w855:dbl)
                        n566 = To Long Integer(number=w855) -> (32bit integer=w854:i32)
                        n567 = Bundle By Name(cluster=w863, "Horizontal"=w854) -> (w852:T1)
                        n568 = local write "right Coords"(w852) -> ()
                        n569 = Unbundle By Name(w852) -> ("Horizontal"=w878:i32)
                        n570 = Unbundle By Name(w852) -> ("Vertical"=w918:i32)
                        n571 = To Double Precision Float(number=w918) -> (double precision float=w912:dbl)
                        n572 = To Double Precision Float(number=w878) -> (double precision float=w903:dbl)
                        n573 = Subtract(x=w903, y=w857) -> (x-y=w868:dbl)
                        n574 = Subtract(x=w912, y=w911) -> (x-y=w867:dbl)
                        n575 = Bundle By Name(cluster=w852, "Horizontal"=w868, "Vertical"=0) -> (w879:T1)
                        n576 = Subtract(x=w907, y=w867) -> (x-y=w910:dbl)
                        n577 = In Range and Coerce(upper limit=w859, x=w868, lower limit=0.0) -> (coerced(x)=w905:dbl)  [unwired: 1 out]
                        n578 = In Range and Coerce(upper limit=w907, x=w910, lower limit=0.0) -> (coerced(x)=w908:dbl)  [unwired: 1 out]
                        n579 = Bundle By Name(cluster=w852, "Horizontal"=w868, "Vertical"=w867) -> (w869:T1)
                        n580 = Divide(x=w905, y=w859) -> (x/y=w901:dbl)
                        n581 = Subtract(x=w919, y=w914) -> (x-y=w917:dbl)
                        n582 = Divide(x=w908, y=w907) -> (x/y=w916:dbl)
                        n583 = Multiply(x=w861, y=w901) -> (x*y=w902:dbl)
                        n584 = Multiply(x=w917, y=w916) -> (x*y=w915:dbl)
                        n585 = call <vilib>:"Draw Point.vi"("picture"=w871, "point(x,y)"=w869, "color(black)"=w853, "pen"=T5 {"Width"=6, "Style"=enum."Solid"}) -> ("new picture"=w870:picture)  [unwired: 5 in]
                        n586 = Bundle By Name(cluster=w852, "Horizontal"=w868, "Vertical"=w877) -> (w876:T1)
                        n587 = property on="Right Graph" class="IntGraph (strict)"() -> ("XScale.Multiplier"=w891:dbl, "XScale.Offset"=w893:dbl, "YScale.Multiplier"=w886:dbl, "YScale.Offset"=w888:dbl)  [unwired: 2 in, 2 out]
                        n588 = Add(x=w902, y=w899) -> (x+y=w883:dbl)
                        n589 = Add(x=w915, y=w914) -> (x+y=w882:dbl)
                        n590 = call <vilib>:"Move Pen.vi"("new position"=w879, "picture"=w870) -> ("new picture"=w881:picture)  [unwired: 3 in]
                        n591 = Subtract(x=w882, y=w888) -> (x-y=w887:dbl)
                        n592 = Subtract(x=w883, y=w893) -> (x-y=w892:dbl)
                        n593 = call <vilib>:"Draw Line.vi"("picture"=w881, "end point"=w876, "color(black)"=w853, "pen"=T5 {"Width"=2, "Style"=enum."Dash"}) -> ("new picture"=w874:picture)  [unwired: 5 in]
                        n594 = Divide(x=w887, y=w886) -> (x/y=w885:dbl)
                        n595 = Divide(x=w892, y=w891) -> (x/y=w890:dbl)
                        n596 = Round To Nearest(number=w885) -> (nearest integer value=w884:dbl)
                        n597 = property on="Property Node" class="IntensityGraph (strict)"(reference=w875, "PlotImages.Front"=w874) -> ()  [unwired: 1 in, 2 out]
                        n598 = Round To Nearest(number=w890) -> (nearest integer value=w889:dbl)
                        n599 = Index Array(array=w896, index (dim 1)=w884, index (dim 2)=w889) -> (element=w865:i32[])  [unwired: 1 in]
                        n600 = local write "right wvf graph"(w865) -> ()
                        n601 = Index Array(array=w896, index (dim 2)=w889) -> (element=w895:i32[][])  [unwired: 2 in]
                        n602 = Transpose 2D Array(2D array=w895) -> (transposed array=w894:i32[][])
                        n603 = local write "Left Graph"(w894) -> ()
                      }
                      event "Y": Value Change {
                        w937 = FALSE
                        # "<-- asymmetry"
                        # "Needed because panel (0,0) is at TOP left rather than bottom left."
                        n604 = event-data() -> ("NewVal"=w935:dbl)  [unwired: 1 in]
                        n605 = local read "right Coords"() -> (w936:T1)
                        n606 = local read "right color"() -> (w929:u32)
                        n607 = control-ref of="Right Graph"() -> (w948:refnum<vi>)
                        n608 = property on="Property Node" class="IntensityGraph (strict)"(reference=w948) -> ("X Scale.Range:Maximum"=w973:dbl, "X Scale.Range:Minimum"=w972:dbl, "Plot Area:Size:Width"=w971:u32, "Plot Area:Position:Left"=w970:i32)  [unwired: 1 in, 2 out]
                        n609 = property on="Property Node" class="IntensityGraph (strict)"(reference=w948) -> ("Y Scale.Range:Maximum"=w989:dbl, "Y Scale.Range:Minimum"=w985:dbl, "Plot Area:Size:Height"=w984:u32, "Plot Area:Position:Top"=w979:i32)  [unwired: 1 in, 2 out]
                        n610 = call "Empty Picture"() -> ("empty picture"=w946:picture)
                        n611 = property on="Property Node" class="IntensityGraph (strict)"(reference=w948, "PlotImages.Front"=w946) -> ("Height"=w950:u32, "PlotImages.Front"=w944:picture)  [unwired: 1 in, 2 out]
                        n612 = To Double Precision Float(number=w970) -> (double precision float=w932:dbl)
                        n613 = To Double Precision Float(number=w979) -> (double precision float=w921:dbl)
                        n614 = To Double Precision Float(number=w971) -> (double precision float=w933:dbl)
                        n615 = To Double Precision Float(number=w984) -> (double precision float=w927:dbl)
                        n616 = Subtract(x=w973, y=w972) -> (x-y=w934:dbl)
                        n617 = Subtract(x=w989, y=w985) -> (x-y=w928:dbl)
                        n618 = Divide(x=w935, y=w928) -> (x/y=w925:dbl)
                        n619 = Subtract(x=1.0, y=w925) -> (x-y=w923:dbl)
                        n620 = Multiply(x=w923, y=w927) -> (x*y=w922:dbl)
                        n621 = Add(x=w922, y=w921) -> (x+y=w926:dbl)
                        n622 = Round To Nearest(number=w926) -> (nearest integer value=w931:dbl)
                        n623 = To Long Integer(number=w931) -> (32bit integer=w930:i32)
                        n624 = Bundle By Name(cluster=w936, "Vertical"=w930) -> (w920:T1)
                        n625 = local write "right Coords"(w920) -> ()
                        n626 = Unbundle By Name(w920) -> ("Horizontal"=w951:i32)
                        n627 = Unbundle By Name(w920) -> ("Vertical"=w988:i32)
                        n628 = To Double Precision Float(number=w988) -> (double precision float=w983:dbl)
                        n629 = To Double Precision Float(number=w951) -> (double precision float=w976:dbl)
                        n630 = Subtract(x=w976, y=w932) -> (x-y=w941:dbl)
                        n631 = Subtract(x=w983, y=w921) -> (x-y=w940:dbl)
                        n632 = Bundle By Name(cluster=w920, "Horizontal"=w941, "Vertical"=0) -> (w952:T1)
                        n633 = Subtract(x=w927, y=w940) -> (x-y=w982:dbl)
                        n634 = In Range and Coerce(upper limit=w933, x=w941, lower limit=0.0) -> (coerced(x)=w978:dbl)  [unwired: 1 out]
                        n635 = In Range and Coerce(upper limit=w927, x=w982, lower limit=0.0) -> (coerced(x)=w980:dbl)  [unwired: 1 out]
                        n636 = Bundle By Name(cluster=w920, "Horizontal"=w941, "Vertical"=w940) -> (w942:T1)
                        n637 = Divide(x=w978, y=w933) -> (x/y=w974:dbl)
                        n638 = Divide(x=w980, y=w927) -> (x/y=w987:dbl)
                        n639 = Multiply(x=w934, y=w974) -> (x*y=w975:dbl)
                        n640 = Multiply(x=w928, y=w987) -> (x*y=w986:dbl)
                        n641 = call <vilib>:"Draw Point.vi"("picture"=w944, "point(x,y)"=w942, "color(black)"=w929, "pen"=T5 {"Width"=6, "Style"=enum."Solid"}) -> ("new picture"=w943:picture)  [unwired: 5 in]
                        n642 = Bundle By Name(cluster=w920, "Horizontal"=w941, "Vertical"=w950) -> (w949:T1)
                        n643 = property on="Right Graph" class="IntGraph (strict)"() -> ("XScale.Multiplier"=w964:dbl, "XScale.Offset"=w966:dbl, "YScale.Multiplier"=w959:dbl, "YScale.Offset"=w961:dbl)  [unwired: 2 in, 2 out]
                        n644 = Add(x=w975, y=w972) -> (x+y=w956:dbl)
                        n645 = Add(x=w986, y=w985) -> (x+y=w955:dbl)
                        n646 = call <vilib>:"Move Pen.vi"("new position"=w952, "picture"=w943) -> ("new picture"=w954:picture)  [unwired: 3 in]
                        n647 = Subtract(x=w955, y=w961) -> (x-y=w960:dbl)
                        n648 = Subtract(x=w956, y=w966) -> (x-y=w965:dbl)
                        n649 = call <vilib>:"Draw Line.vi"("picture"=w954, "end point"=w949, "color(black)"=w929, "pen"=T5 {"Width"=2, "Style"=enum."Dash"}) -> ("new picture"=w947:picture)  [unwired: 5 in]
                        n650 = Divide(x=w960, y=w959) -> (x/y=w958:dbl)
                        n651 = Divide(x=w965, y=w964) -> (x/y=w963:dbl)
                        n652 = Round To Nearest(number=w958) -> (nearest integer value=w957:dbl)
                        n653 = property on="Property Node" class="IntensityGraph (strict)"(reference=w948, "PlotImages.Front"=w947) -> ()  [unwired: 1 in, 2 out]
                        n654 = Round To Nearest(number=w963) -> (nearest integer value=w962:dbl)
                        n655 = Index Array(array=w969, index (dim 1)=w957, index (dim 2)=w962) -> (element=w938:i32[])  [unwired: 1 in]
                        n656 = local write "right wvf graph"(w938) -> ()
                        n657 = Index Array(array=w969, index (dim 2)=w962) -> (element=w968:i32[][])  [unwired: 2 in]
                        n658 = Transpose 2D Array(2D array=w968) -> (transposed array=w967:i32[][])
                        n659 = local write "Left Graph"(w967) -> ()
                      }
                      event "graph real ratio?": Value Change {
                        w990 = FALSE
                        n660 = event-data() -> ("NewVal"=w992:bool)  [unwired: 1 in, 2 out]
                        n661 = control-ref of="Right Graph"() -> (w991:refnum<vi>)
                        n662 = case shown="True" w992 {
                          tunnel: w991 -> [w995 w999]
                          frame False {
                            n663 = property on="Left Graph" class="IntGraph (strict)"() -> ("YScale.Maximum"=w993:dbl)  [unwired: 2 in, 2 out]
                            n664 = property on="Scan Length (mm)" class="DigNum (strict)"() -> ("Value"=w994:dbl)  [unwired: 2 in, 2 out]
                            n665 = property class="IntGraph (strict)"(reference=w995, "YScale.Maximum"=w993, "XScale.Maximum"=w994) -> ()  [unwired: 1 in, 2 out]
                          }
                          frame True {
                            n666 = property class="IntGraph (strict)"(reference=w999) -> ("XScale.Maximum"=w998:dbl)  [unwired: 1 in, 2 out]
                            n667 = property on="Left Graph" class="IntGraph (strict)"() -> ("YScale.Maximum"=w996:dbl)  [unwired: 2 in, 2 out]
                            n668 = Less?(x=w998, y=w996) -> (x < y?=w997:bool)
                            n669 = case shown="False" w997 {
                              tunnel: w999 -> [w1003 w1005]
                              frame False {
                                n670 = property class="IntGraph (strict)"(reference=w1003, "YScale.ScaleFit"=u8 0 ("Y Scale.Scale Fit")) -> (reference out=w1002:refnum<vi>, "XScale.Maximum"=w1000:dbl)  [unwired: 1 in, 1 out]
                                n671 = property class="IntGraph (strict)"(reference=w1002, "YScale.Maximum"=w1000) -> ()  [unwired: 1 in, 2 out]
                              }
                              frame True {
                                n672 = property class="IntGraph (strict)"(reference=w1005, "XScale.ScaleFit"=u8 0 ("Y Scale.Scale Fit")) -> (reference out=w1007:refnum<vi>, "YScale.Maximum"=w1004:dbl)  [unwired: 1 in, 1 out]
                                n673 = property class="IntGraph (strict)"(reference=w1007, "XScale.Maximum"=w1004) -> ()  [unwired: 1 in, 2 out]
                              }
                            }
                          }
                        }
                      }
                      event "Shut Down": Mouse Down {
                        n674 = event-data() -> ()  [unwired: 1 in, 8 out]
                        n675 = local read "scanned?"() -> (w1009:bool)
                        n676 = case shown="True" w1009 {
                          tunnel: [TRUE w1012] -> w1010
                          frame False {
                          }
                          frame True {
                            n677 = global read "applicationControl.vi" "Saved?"() -> (w1013:bool)
                            n678 = case shown="False" w1013 {
                              tunnel: [w1014 TRUE ("Shut Down")] -> w1012
                              frame False {
                                n679 = Two Button Dialog(message="Haven't save the file, still shut down?", 1:"Cancel" ("F button name (\"Cancel\")"), 2:"Shut down without saving" ("T button name (\"OK\")")) -> (T button?=w1015:bool)
                                n680 = case shown="False" w1015 {
                                tunnel: [FALSE TRUE] -> w1014
                                frame False {
                                }
                                frame True {
                                }
                                }
                              }
                              frame True {
                              }
                            }
                          }
                        }
                      }
                      event "Wipe and Quit": Mouse Down {
                        n681 = event-data() -> ()  [unwired: 1 in, 8 out]
                        n682 = global read "applicationControl.vi" "Saved?"() -> (w1024:bool)
                        n683 = case shown="True" w1024 {
                          tunnel: [w1025 TRUE ("Shut Down")] -> w1023
                          frame False {
                            n684 = Two Button Dialog(message="Haven't save the file, wipe data?", 1:"Cancel" ("F button name (\"Cancel\")"), 2:"Start again without saving" ("T button name (\"OK\")")) -> (T button?=w1026:bool)
                            n685 = case shown="False" w1026 {
                              tunnel: [FALSE TRUE] -> w1025
                              frame False {
                              }
                              frame True {
                              }
                            }
                          }
                          frame True {
                          }
                        }
                      }
                      event "Read File": Value Change {
                        w1035 = FALSE
                        n686 = event-data() -> ()  [unwired: 1 in, 6 out]
                        n687 = local read "Read mode"() -> (w1034:bool)
                        n688 = case shown="False" w1034 {
                          tunnel: [w1081 TRUE] -> w1033
                          frame False {
                            n689 = global read "applicationControl.vi" "Saved?"() -> (w1082:bool)
                            n690 = case shown="False" w1082 {
                              tunnel: [w1083 TRUE ("Shut Down")] -> w1081
                              frame False {
                                n691 = Two Button Dialog(message="Haven't save the file, wipe data?", 1:"Cancel" ("F button name (\"Cancel\")"), 2:"Load new data \nwithout saving current one" ("T button name (\"OK\")")) -> (T button?=w1084:bool)
                                n692 = case shown="True" w1084 {
                                tunnel: [FALSE TRUE] -> w1083
                                frame False {
                                }
                                frame True {
                                }
                                }
                              }
                              frame True {
                              }
                            }
                          }
                          frame True {
                          }
                        }
                        n693 = case shown="True" w1033 {
                          frame False {
                          }
                          frame True {
                            n694 = flat-sequence {
                              tunnel: [w1051] -> w1043
                              tunnel: [w1050] -> w1042
                              tunnel: [w1049] -> w1041
                              tunnel: [w1048] -> w1040
                              tunnel: [w1047] -> w1039
                              tunnel: [w1046] -> w1038
                              tunnel: [w1045] -> w1037
                              tunnel: [w1044] -> w1036
                              tunnel: w1043 -> [w1076]
                              tunnel: w1042 -> [w1074]
                              tunnel: w1041 -> [w1073]
                              tunnel: w1040 -> [w1072]
                              tunnel: w1039 -> [w1067]
                              tunnel: w1038 -> [w1062]
                              tunnel: w1037 -> [w1068]
                              tunnel: w1036 -> [w1065]
                              frame #0 {
                                n695 = local read "Path"() -> (w1052:path)
                                n696 = control-ref of="HSS (MHz)"() -> (w1050:refnum<vi>)
                                n697 = control-ref of="Left Graph"() -> (w1046:refnum<vi>)
                                n698 = control-ref of="Right Graph"() -> (w1047:refnum<vi>)
                                n699 = control-ref of="VSS (s)"() -> (w1049:refnum<vi>)
                                n700 = call "readTiff.vi"("file (use dialog)"=w1052) -> ("Vss"=w1048:sgl, "HSS"=w1051:u32, "imageHeight"=w1044:i32, "imageWidth"=w1045:i32)  [unwired: 7 in]
                              }
                              frame #1 {
                                w1064 = 0.0 ("X Scale.Offset and Multiplier:Offset")
                                n701 = global read "imageSettings.vi" "Exposure Time (s)"() -> (w1078:sgl)
                                n702 = global read "imageSettings.vi" "realXDimension"() -> (w1080:dbl)
                                n703 = global read "imageSettings.vi" "stepLength"() -> (w1079:u32)
                                n704 = Format Value(format string="%.3f", value (0)=w1072) -> (output string=w1070:string)  [unwired: 1 in]
                                n705 = Number To Decimal String(number=w1076) -> (decimal integer string=w1075:string)  [unwired: 1 in]
                                n706 = property class="Ring (strict)"(reference=w1073, "RingText.Text"=w1070) -> ()  [unwired: 1 in, 2 out]
                                n707 = property class="Ring (strict)"(reference=w1074, "RingText.Text"=w1075) -> ()  [unwired: 1 in, 2 out]
                                n708 = To Double Precision Float(number=w1079) -> (double precision float=w1077:dbl)
                                n709 = local write "Scan Length (mm)"(w1080) -> ()
                                n710 = local write "Exposure Time (s)"(w1078) -> ()
                                n711 = local write "Scan Step (um)"(w1077) -> ()
                                n712 = global read "imageSettings.vi" "specArray"() -> (w1061:sgl[])
                                n713 = global read "imageSettings.vi" "realYDimension"() -> (w1053:dbl)
                                n714 = global read "imageSettings.vi" "realXDimension"() -> (w1069:dbl)
                                n715 = Array Size(array=w1061) -> (size(s)=w1060:i32)
                                n716 = Array Max & Min(array=w1061) -> (max value=w1058:sgl, min value=w1057:sgl)  [unwired: 2 out]
                                n717 = Subtract(x=w1058, y=w1057) -> (x-y=w1059:sgl)
                                n718 = Divide(x=w1059, y=w1060) -> (x/y=w1056:sgl)
                                n719 = property on="right wvf graph" class="WFGraph (strict)"("XScale.Multiplier"=w1056, "XScale.Offset"=w1057) -> ()  [unwired: 2 in, 2 out]
                                n720 = property on="left wvf graph" class="WFGraph (strict)"("XScale.Multiplier"=w1056, "XScale.Offset"=w1057) -> ()  [unwired: 2 in, 2 out]
                                n721 = Divide(x=w1053, y=w1065) -> (x/y=w1063:dbl)
                                n722 = Divide(x=w1069, y=w1068) -> (x/y=w1066:dbl)
                                n723 = property class="IntGraph (strict)"(reference=w1062, "YScale.Multiplier"=w1063, "YScale.Offset"=w1064, "XScale.Multiplier"=w1056, "XScale.Offset"=w1057) -> (reference out=w1054:refnum<vi>)  [unwired: 1 in, 1 out]
                                n724 = property class="IntGraph (strict)"(reference=w1067, "XScale.Multiplier"=w1066, "XScale.Offset"=w1064, "YScale.Multiplier"=w1063, "YScale.Offset"=w1064) -> (reference out=w1055:refnum<vi>)  [unwired: 1 in, 1 out]
                                n725 = property class="IntGraph (strict)"(reference=w1055, "YScale.Maximum"=w1053) -> ()  [unwired: 1 in, 2 out]
                                n726 = property class="IntGraph (strict)"(reference=w1054, "YScale.Maximum"=w1053) -> ()  [unwired: 1 in, 2 out]
                              }
                            }
                          }
                        }
                      }
                      event "Save File": Value Change {
                        w1092 = FALSE
                        n727 = event-data() -> ()  [unwired: 1 in, 3 out]
                        n728 = local read "Save File"() -> (w1093:bool)
                        n729 = case shown="True" w1093 {
                          frame False {
                          }
                          frame True {
                            n730 = global write "applicationControl.vi" "Saved?"(TRUE ("Saved?")) -> ()
                            n731 = call "saveFile.vi"("path"="Path") -> ()  [unwired: 11 in]
                          }
                        }
                      }
                      event Timeout {
                        w1096 = FALSE
                        n732 = event-data() -> ()  [unwired: 1 in, 3 out]
                        n733 = local read "X"() -> (w1098:dbl)
                        n734 = local read "Y"() -> (w1097:dbl)
                      }
                    }
                    n735 = Negate(x=w655) -> (-x=w654:dbl)
                    n736 = Subtract(x="Wavelength slide", y=w656) -> (x-y=w667:dbl)
                    n737 = global read "configDB.vi" "sensorStart"() -> (w636:i32)
                    n738 = Multiply(x=w637, y=w654) -> (x*y=w659:dbl)
                    n739 = Add(x=w667, y=w659) -> (x+y=w660:dbl)
                    n740 = Divide(x=w660, y=w654) -> (x/y=w666:dbl)
                    n741 = Increment(x=w636) -> (x+1=w635:i32)
                    n742 = Round To Nearest(number=w666) -> (nearest integer value=w657:dbl)
                    n743 = Array Size(array=w665) -> (size(s)=w676:i32[])
                    n744 = Subtract(x=w657, y=w635) -> (x-y=w658:dbl)
                    n745 = Less?(x="Bandwidth (Frame)", y=w658) -> (x < y?=w672:bool)
                    n746 = Not Equal?(x="Bandwidth (Frame)", y=0.0) -> (x != y?=w671:bool)
                    n747 = Index Array(array=w676, index=2) -> (element=w674:i32)
                    n748 = Index Array(array=w676, index=1) -> (element=w673:i32)
                    n749 = And(x=w672, y=w671) -> (x .and. y?=w670:bool)
                    n750 = Multiply(x=2.0, y="Bandwidth (Frame)") -> (x*y=w678:dbl)
                    n751 = event shown="[0] Timeout" {
                      selector: _ -> [_ _]
                      dyn-events: _ -> [_ _]
                      timeout: 10 -> [_ _]
                      tunnel: [w760 w768] -> w682
                      tunnel: w658 -> [_ w761]
                      tunnel: "Bandwidth (Frame)" -> [_ w767]
                      tunnel: w665 -> [_ w766]
                      tunnel: w678 -> [_ w765]
                      tunnel: w674 -> [_ w764]
                      tunnel: w673 -> [_ w763]
                      tunnel: w670 -> [_ w762]
                      event Timeout {
                        n752 = event-data() -> ()  [unwired: 1 in, 3 out]
                        n753 = local read "Right Graph"() -> (w760:i32[][])
                      }
                      event "Bandwidth (Frame)", "Wavelength slide": Value Change {
                        n754 = event-data() -> ()  [unwired: 1 in, 6 out]
                        n755 = case shown="True" w762 {
                          tunnel: w761 -> [w771 w780]
                          tunnel: w766 -> [w770 w781]
                          tunnel: w765 -> [_ w772]
                          tunnel: [w769 w779] -> w768
                          tunnel: w767 -> [_ w778]
                          tunnel: w764 -> [_ w775]
                          tunnel: w763 -> [_ w774]
                          frame False {
                            n756 = Index Array(array=w770, index (dim 0)=w771) -> (element=w769:i32[][])  [unwired: 2 in]
                          }
                          frame True {
                            n757 = Initialize Array(0 ("element"), w774, w775) -> (w776:i32[][])
                            n758 = for {
                              N: w772 -> [_]
                              tunnel: w781 -> [w790]
                              shift-right: [w788] -> w773
                              shift-left: w776 -> [w785]
                              tunnel: w780 -> [w784]
                              tunnel: w778 -> [w783]
                              i -> [w789]
                              n759 = Subtract(x=w784, y=w783) -> (x-y=w782:dbl)
                              n760 = Add(x=w789, y=w782) -> (x+y=w787:dbl)
                              n761 = Index Array(array=w790, index (dim 0)=w787) -> (element=w786:i32[][])  [unwired: 2 in]
                              n762 = Add ("Add.vi")(x=w786, y=w785) -> (x+y=w788:i32[][])
                            }
                            n763 = Divide(x=w773, y=w772) -> (x/y=w779:dbl[][])
                          }
                        }
                      }
                    }
                    n764 = local read "left wvf color 3"() -> (w633:u32)
                    n765 = control-ref of="Left Graph"() -> (w640:refnum<vi>)
                    n766 = local write "Y"(w630) -> ()
                    n767 = local write "X"(w631) -> ()
                    n768 = local read "left WaveMouse"() -> (w647:i32)
                    n769 = local read "right WaveMouse 2"() -> (w646:i32)
                    n770 = control-ref of="right wvf graph"() -> (w650:refnum<vi>)
                    n771 = local read "right wvf color 4"() -> (w632:u32)
                    n772 = control-ref of="left wvf graph"() -> (w651:refnum<vi>)
                    n773 = property on="Property Node" class="IntGraph (strict)"(reference=w640) -> ("Value"=w653:i32[][])  [unwired: 1 in, 2 out]
                    n774 = case shown="\"Horizontal\", Default" "Line Profile" {
                      tunnel: w653 -> [w691 w719]
                      tunnel: [w690 w724] -> w652
                      tunnel: "line avg?" -> [w692 w723]
                      tunnel: w640 -> [w687 w721]
                      tunnel: "Line Profile" -> [w689 w722]
                      tunnel: "left Coords" -> [w688 w720]
                      tunnel: "left color 2" -> [w686 w718]
                      tunnel: [w685 w717] -> w629
                      frame "Vertical" {
                        n775 = case shown="False" w692 {
                          tunnel: w691 -> [w702 w709]
                          tunnel: [w701 w707] -> w690
                          tunnel: w687 -> [w693 w706]
                          tunnel: w689 -> [w703 _]
                          tunnel: w688 -> [w700 _]
                          tunnel: w686 -> [w699 _]
                          tunnel: [w694 0] -> w685
                          frame False {
                            n776 = property class="IntGraph (strict)"(reference=w693) -> ("XScale.Multiplier"=w697:dbl, "XScale.Offset"=w695:dbl)  [unwired: 1 in, 2 out]
                            n777 = call "drawIntensityGraph.vi"("color(black)"=w699, "Combo Box"=w703, "Coords"=w700, "Left Graph 2"=w693) -> ("x"=w698:i32)  [unwired: 6 in, 1 out]
                            n778 = Index Array(array=w702, index (col)=w698) -> (element=w701:i32[])  [unwired: 1 in]
                            n779 = Multiply(x=w698, y=w697) -> (x*y=w696:dbl)
                            n780 = Add(x=w696, y=w695) -> (x+y=w694:dbl)
                          }
                          frame True {
                            n781 = call "Empty Picture"() -> ("empty picture"=w705:picture)
                            n782 = for {
                              N: 512 -> [_]
                              tunnel: w709 -> [w715]
                              tunnel: [w711] -> w707 mode=indexing
                              i -> [w710]
                              n783 = Index Array(array=w715, index (row)=w710) -> (element=w714:i32[])  [unwired: 1 in]
                              n784 = Add Array Elements(numeric array=w714) -> (sum=w713:i32)
                              n785 = Divide(x=w713, y=384) -> (x/y=w711:dbl)
                            }
                            n786 = property on="Property Node" class="IntGraph (strict)"(reference=w706, "PlotImages.Front"=w705) -> ()  [unwired: 1 in, 2 out]
                          }
                        }
                        n787 = property on="left profie location" class="DigNum (strict)"("Caption.Text"="Wavelength" ("Label.Text")) -> ()  [unwired: 2 in, 2 out]
                      }
                      frame "Horizontal", Default {
                        n788 = case shown="False" w723 {
                          tunnel: w719 -> [w734 w740]
                          tunnel: [w733 w739] -> w724
                          tunnel: w722 -> [w735 _]
                          tunnel: w721 -> [w730 w737]
                          tunnel: w720 -> [w732 _]
                          tunnel: w718 -> [w731 _]
                          tunnel: [w725 0] -> w717
                          frame False {
                            n789 = property class="IntGraph (strict)"(reference=w730) -> ("YScale.Multiplier"=w729:dbl, "YScale.Offset"=w727:dbl)  [unwired: 1 in, 2 out]
                            n790 = call "drawIntensityGraph.vi"("color(black)"=w731, "Combo Box"=w735, "Coords"=w732, "Left Graph 2"=w730) -> ("y"=w726:i32)  [unwired: 6 in, 1 out]
                            n791 = Index Array(array=w734, index (row)=w726) -> (element=w733:i32[])  [unwired: 1 in]
                            n792 = Multiply(x=w726, y=w729) -> (x*y=w728:dbl)
                            n793 = Add(x=w728, y=w727) -> (x+y=w725:dbl)
                          }
                          frame True {
                            n794 = call "Empty Picture"() -> ("empty picture"=w738:picture)
                            n795 = for {
                              N: 384 -> [_]
                              tunnel: w740 -> [w747]
                              tunnel: [w742] -> w739 mode=indexing
                              i -> [w746]
                              n796 = Index Array(array=w747, index (col)=w746) -> (element=w745:i32[])  [unwired: 1 in]
                              n797 = Add Array Elements(numeric array=w745) -> (sum=w744:i32)
                              n798 = Divide(x=w744, y=512) -> (x/y=w742:dbl)
                            }
                            n799 = property on="Property Node" class="IntGraph (strict)"(reference=w737, "PlotImages.Front"=w738) -> ()  [unwired: 1 in, 2 out]
                          }
                        }
                        n800 = property on="left profie location" class="DigNum (strict)"("Caption.Text"="Y" ("Label.Text")) -> ()  [unwired: 2 in, 2 out]
                      }
                    }
                    n801 = Or(x=w643, y=w642) -> (x .or. y?=w669:bool)
                    n802 = call "waveformGraphDraw.vi"("color(black)"=w633, "WaveMouse 2"=w647, "right wvf graph 2"=w651) -> ("Wavelength 2"=w648:dbl, "Intensity 2"=w649:i32)  [unwired: 7 in]
                    n803 = call "waveformGraphDraw.vi"("color(black)"=w632, "WaveMouse 2"=w646, "right wvf graph 2"=w650) -> ("Wavelength 2"=w644:dbl, "Intensity 2"=w645:i32)  [unwired: 7 in]
                    n804 = local write "left profie location"(w629) -> ()
                    n805 = local write "left Wavelength"(w648) -> ()
                    n806 = local write "Shut Down"(w642) -> ()
                    n807 = local write "right Wavelength"(w644) -> ()
                    n808 = local write "Right Graph"(w682) -> ()
                    n809 = local write "Intensity"(w649) -> ()
                    n810 = local write "Intensity 2"(w645) -> ()
                    n811 = local write "left wvf graph"(w652) -> ()
                  }
                }
              }
              frame #2 {
                w1101 = FALSE ("Visible")
                w1100 = T4."Enabled" ("Disabled")
                w1099 = T4."Disabled and Grayed Out" ("Disabled")
                n812 = property on="Read mode" class="Bool (strict)"("DisabledEnum"=w1100) -> ()  [unwired: 2 in, 2 out]
                n813 = property on="Go Origin" class="Bool"("DisabledEnum"=w1100) -> ()  [unwired: 2 in, 2 out]
                n814 = property on="Set Origin" class="Bool"("DisabledEnum"=w1100) -> ()  [unwired: 2 in, 2 out]
                n815 = property on="go right Button" class="Bool"("DisabledEnum"=w1100) -> ()  [unwired: 2 in, 2 out]
                n816 = property on="Set Temperature" class="DigNum (strict)"("DisabledEnum"=w1100) -> ()  [unwired: 2 in, 2 out]
                n817 = local write "graph real ratio?"(w1101) -> ()
                n818 = property on="X" class="DigNum (strict)"("Visible"=w1101) -> ()  [unwired: 2 in, 2 out]
                n819 = property on="Y" class="DigNum (strict)"("Visible"=w1101) -> ()  [unwired: 2 in, 2 out]
                n820 = property on="Read File" class="Bool (strict)"("DisabledEnum"=w1099) -> ()  [unwired: 2 in, 2 out]
                n821 = property on="right wvf graph" class="WFGraph (strict)"("Value"=i32[] [] ("right wvf graph")) -> ()  [unwired: 2 in, 2 out]
                n822 = global write "imageSettings.vi" "backgroundExist"(w1101) -> ()
                n823 = property on="Scan Step (um)" class="DigNum (strict)"("DisabledEnum"=w1100) -> ()  [unwired: 2 in, 2 out]
                n824 = global write "applicationControl.vi" "Saved?"(w1101) -> ()
                n825 = property on="go left Button" class="Bool"("DisabledEnum"=w1100) -> ()  [unwired: 2 in, 2 out]
                n826 = local write "scanned?"(w1101) -> ()
                n827 = property on="right wvf graph" class="WFGraph (strict)"("Caption.Text"="On Sensor Image Average") -> ()  [unwired: 2 in, 2 out]
                n828 = property on="graph real ratio?" class="Bool (strict)"("Visible"=w1101) -> ()  [unwired: 2 in, 2 out]
                n829 = global write "imageSettings.vi" "referenceExist"(w1101) -> ()
                n830 = property on="Shutter Control" class="Enum (strict)"("DisabledEnum"=w1100) -> ()  [unwired: 2 in, 2 out]
                n831 = property on="Exposure Time (s)" class="DigNum (strict)"("DisabledEnum"=w1100) -> ()  [unwired: 2 in, 2 out]
                n832 = property on="VSS (s)" class="Ring (strict)"("DisabledEnum"=w1100) -> ()  [unwired: 2 in, 2 out]
                n833 = property on="Path" class="Path"("DisabledEnum"=w1099) -> ()  [unwired: 2 in, 2 out]
                n834 = property on="Scan Start" class="Bool"("DisabledEnum"=w1100) -> ()  [unwired: 2 in, 2 out]
                n835 = property on="Wipe and Quit" class="Bool"("DisabledEnum"=w1099) -> ()  [unwired: 2 in, 2 out]
                n836 = call "Empty Picture"() -> ("empty picture"=w1105:picture)
                n837 = property on="OM" class="Bool (strict)"("DisabledEnum"=w1100) -> ()  [unwired: 2 in, 2 out]
                n838 = property on="Bandwidth (Frame)" class="DigNum (strict)"("Visible"=w1101) -> ()  [unwired: 2 in, 2 out]
                n839 = property on="Background" class="Bool"("DisabledEnum"=w1100) -> ()  [unwired: 2 in, 2 out]
                n840 = property on="Wavelength slide" class="Slide (strict)"("Visible"=w1101) -> ()  [unwired: 2 in, 2 out]
                n841 = property on="Reference" class="Bool"("DisabledEnum"=w1100) -> ()  [unwired: 2 in, 2 out]
                n842 = property on="Save File" class="Bool (strict)"("DisabledEnum"=w1099) -> ()  [unwired: 2 in, 2 out]
                n843 = property on="left wvf graph" class="WFGraph (strict)"("PlotImages.Front"=w1105) -> ()  [unwired: 2 in, 2 out]
                n844 = invoke on="Right Graph" class="IntGraph (strict)" method="Reinit To Default"() -> ()  [unwired: 3 in, 3 out]
                n845 = invoke on="Left Graph" class="IntGraph (strict)" method="Reinit To Default"() -> ()  [unwired: 3 in, 3 out]
                n846 = invoke on="left wvf graph" class="WFGraph (strict)" method="Reinit To Default"() -> ()  [unwired: 3 in, 3 out]
                n847 = property on="right wvf graph" class="WFGraph (strict)"("PlotImages.Front"=w1105) -> ()  [unwired: 2 in, 2 out]
                n848 = property on="Go back after scan" class="Bool (strict)"("DisabledEnum"=w1100) -> ()  [unwired: 2 in, 2 out]
                n849 = property on="Right Graph" class="IntGraph (strict)"("PlotImages.Front"=picture data[5B] ("Plot Images:Front"), "YScale.ScaleFit"=u8 1 ("Y Scale.Scale Fit")) -> ()  [unwired: 2 in, 2 out]
                n850 = property on="Live View" class="Bool (strict)"("DisabledEnum"=w1100) -> ()  [unwired: 2 in, 2 out]
                n851 = property on="Take shot" class="Bool (strict)"("DisabledEnum"=w1100) -> ()  [unwired: 2 in, 2 out]
                n852 = property on="HSS (MHz)" class="Ring (strict)"("DisabledEnum"=w1100) -> ()  [unwired: 2 in, 2 out]
                n853 = property on="Scan Length (mm)" class="DigNum (strict)"("DisabledEnum"=w1100) -> ()  [unwired: 2 in, 2 out]
                n854 = property on="Step length (um)" class="DigNum (strict)"("DisabledEnum"=w1100) -> ()  [unwired: 2 in, 2 out]
                n855 = invoke on="Read mode" class="Bool (strict)" method="Reinit To Default"() -> ()  [unwired: 3 in, 3 out]
              }
            }
          }
        }
      }
      n856 = global read "configDB.vi" "floatingDigits"() -> (w53:i32)
      n857 = Negate(x=w53) -> (-x=w51:i32)
      n858 = Power Of 10(x=w51) -> (10^x=w52:dbl)
      n859 = while {
        tunnel: w53 -> [w57]
        tunnel: w52 -> [w56]
        stop <- w58 stop-if-true
        n860 = Add(x=0, y=w57) -> (x+y=w55:i32)
        n861 = event shown="[8] \"left profie location\": Value Change" {
          selector: _ -> [_ _ _ _ _ _ _ _ _ _ _ _]
          dyn-events: _ -> [_ _ _ _ _ _ _ _ _ _ _ _]
          timeout: 10 -> [_ _ _ _ _ _ _ _ _ _ _ _]
          tunnel: w55 -> [_ _ _ _ _ _ _ _ _ w162 _ _]
          tunnel: w56 -> [_ _ _ _ _ _ _ _ _ w161 _ _]
          event Timeout {
            n862 = event-data() -> ()  [unwired: 1 in, 3 out]
          }
          event "right wvf graph": Mouse Down {
            n863 = event-data() -> ("Coords.Horizontal"=w60:i32)  [unwired: 1 in, 7 out]
            n864 = local write "right WaveMouse 2"(w60) -> ()
            n865 = control-ref of="right wvf graph"() -> (w61:refnum<vi>)
            n866 = call "Empty Picture"() -> ("empty picture"=w62:picture)
            n867 = property class="WFGraph (strict)"(reference=w61, "PlotImages.Front"=w62) -> ()  [unwired: 1 in, 2 out]
          }
          event "right Wavelength": Value Change {
            n868 = event-data() -> ("NewVal"=w73:dbl)  [unwired: 1 in, 4 out]
            n869 = control-ref of="right wvf graph"() -> (w77:refnum<vi>)
            n870 = property class="WFGraph (strict)"(reference=w77) -> (reference out=w76:refnum<vi>, "XScale.Maximum"=w75:dbl, "XScale.Minimum"=w63:dbl, "Width"=w71:u32, "Plot Bounds"=w70:T13)  [unwired: 1 in, 1 out]
            n871 = Subtract(x=w73, y=w63) -> (x-y=w64:dbl)
            n872 = Unbundle By Name(w70) -> ("Left"=w68:i16)
            n873 = Subtract(x=w75, y=w63) -> (x-y=w74:dbl)
            n874 = Divide(x=w64, y=w74) -> (x/y=w72:dbl)
            n875 = Multiply(x=w71, y=w72) -> (x*y=w69:dbl)
            n876 = Add(x=w69, y=w68) -> (x+y=w67:dbl)
            n877 = call "Empty Picture"() -> ("empty picture"=w78:picture)
            n878 = property class="WFGraph (strict)"(reference=w76, "PlotImages.Front"=w78) -> ()  [unwired: 1 in, 2 out]
            n879 = Round To Nearest(number=w67) -> (nearest integer value=w66:dbl)
            n880 = To Long Integer(number=w66) -> (32bit integer=w65:i32)
            n881 = local write "right WaveMouse 2"(w65) -> ()
          }
          event "left Wavelength": Value Change {
            n882 = event-data() -> ("NewVal"=w89:dbl)  [unwired: 1 in, 4 out]
            n883 = control-ref of="left wvf graph"() -> (w93:refnum<vi>)
            n884 = property class="WFGraph (strict)"(reference=w93) -> (reference out=w92:refnum<vi>, "XScale.Maximum"=w91:dbl, "XScale.Minimum"=w79:dbl, "Width"=w87:u32, "Plot Bounds"=w86:T13)  [unwired: 1 in, 1 out]
            n885 = Subtract(x=w89, y=w79) -> (x-y=w80:dbl)
            n886 = Unbundle By Name(w86) -> ("Left"=w84:i16)
            n887 = Subtract(x=w91, y=w79) -> (x-y=w90:dbl)
            n888 = Divide(x=w80, y=w90) -> (x/y=w88:dbl)
            n889 = Multiply(x=w87, y=w88) -> (x*y=w85:dbl)
            n890 = Add(x=w85, y=w84) -> (x+y=w83:dbl)
            n891 = call "Empty Picture"() -> ("empty picture"=w94:picture)
            n892 = property class="WFGraph (strict)"(reference=w92, "PlotImages.Front"=w94) -> ()  [unwired: 1 in, 2 out]
            n893 = Round To Nearest(number=w83) -> (nearest integer value=w82:dbl)
            n894 = To Long Integer(number=w82) -> (32bit integer=w81:i32)
            n895 = local write "left WaveMouse"(w81) -> ()
          }
          event "left wvf graph": Mouse Down {
            n896 = event-data() -> ("Coords.Horizontal"=w95:i32)  [unwired: 1 in, 7 out]
            n897 = local write "left WaveMouse"(w95) -> ()
            n898 = call "Empty Picture"() -> ("empty picture"=w96:picture)
            n899 = property on="left wvf graph" class="WFGraph (strict)"("PlotImages.Front"=w96) -> ()  [unwired: 2 in, 2 out]
          }
          event "left graph scale": Value Change {
            n900 = event-data() -> ("NewVal"=w98:bool)  [unwired: 1 in, 5 out]
            n901 = case shown="True" w98 {
              tunnel: [0 2] -> w97
              frame False {
              }
              frame True {
              }
            }
            n902 = property on="Left Graph" class="IntGraph (strict)"("ZScale.ScaleFit"=w97) -> ()  [unwired: 2 in, 2 out]
          }
          event "right graph scale 2": Value Change {
            n903 = event-data() -> ("NewVal"=w102:bool)  [unwired: 1 in, 5 out]
            n904 = case shown="True" w102 {
              tunnel: [0 2] -> w101
              frame False {
              }
              frame True {
              }
            }
            n905 = property on="Right Graph" class="IntGraph (strict)"("ZScale.ScaleFit"=w101) -> ()  [unwired: 2 in, 2 out]
          }
          event "Left Graph": Mouse Down {
            n906 = event-data() -> ("Coords"=w105:T1)  [unwired: 1 in]
            n907 = local write "left Coords"(w105) -> ()
          }
          event "left profie location": Value Change {
            n908 = event-data() -> ("NewVal"=w108:dbl, "OldVal"=w107:dbl)  [unwired: 1 in]
            n909 = control-ref of="Left Graph"() -> (w110:refnum<vi>)
            n910 = local read "Line Profile"() -> (w111:string)
            n911 = Greater?(x=w108, y=w107) -> (0:w106:bool)
            n912 = case shown="\"Vertical\", Default" w111 {
              tunnel: w110 -> [w133 w159]
              tunnel: w108 -> [w132 w156]
              tunnel: [w121 w158] -> w109
              tunnel: w106 -> [w115 _]
              frame "Vertical", Default {
                n913 = property class="IntGraph (strict)"(reference=w133) -> ("XScale.Maximum"=w131:dbl, "XScale.Minimum"=w130:dbl)  [unwired: 1 in, 2 out]
                n914 = property class="IntGraph (strict)"(reference=w133) -> ("Width"=w126:u32, "Plot Bounds"=w123:T13)  [unwired: 1 in, 2 out]
                n915 = To Double Precision Float(number=w126) -> (double precision float=w119:dbl)
                n916 = Subtract(x=w132, y=w130) -> (x-y=w129:dbl)
                n917 = Unbundle By Name(w123) -> ("Left"=w124:i16)
                n918 = Subtract(x=w131, y=w130) -> (x-y=w128:dbl)
                n919 = local read "left Coords"() -> (w117:T1)
                n920 = Divide(x=w129, y=w128) -> (x/y=w127:dbl)
                n921 = Multiply(x=w127, y=w119) -> (x*y=w125:dbl)
                n922 = To Double Precision Float(number=w124) -> (double precision float=w118:dbl)
                n923 = Add(x=w125, y=w118) -> (x+y=w122:dbl)
                n924 = Round To Nearest(number=w122) -> (nearest integer value=w120:dbl)
                n925 = To Long Integer(number=w120) -> (32bit integer=w113:i32)
                n926 = Unbundle By Name(w117) -> ("Horizontal"=w112:i32)
                n927 = Less Or Equal?(x=w113, y=w112) -> (x <= y?=w116:bool)
                n928 = case shown="True" w116 {
                  tunnel: w115 -> [_ w138]
                  tunnel: w113 -> [w134 w137]
                  tunnel: [w134 w136] -> w114
                  tunnel: w112 -> [_ w135]
                  frame False {
                  }
                  frame True {
                    n929 = case shown="False" w138 {
                      tunnel: w137 -> [w139 _]
                      tunnel: [w139 w141] -> w136
                      tunnel: w135 -> [_ w140]
                      frame False {
                      }
                      frame True {
                        n930 = Increment(x=w140) -> (x+1=w141:i32)
                      }
                    }
                  }
                }
                n931 = Bundle By Name(cluster=w117, "Horizontal"=w114) -> (w121:T1)
              }
              frame "Horizontal" {
                n932 = property class="IntGraph (strict)"(reference=w159) -> ("YScale.Maximum"=w155:dbl, "YScale.Minimum"=w154:dbl)  [unwired: 1 in, 2 out]
                n933 = property class="IntGraph (strict)"(reference=w159) -> ("Height"=w149:u32, "Plot Bounds"=w160:T13)  [unwired: 1 in, 2 out]
                n934 = Subtract(x=w155, y=w154) -> (x-y=w153:dbl)
                n935 = Unbundle By Name(w160) -> ("Top"=w146:i16)
                n936 = Divide(x=w156, y=w153) -> (x/y=w152:dbl)
                n937 = To Double Precision Float(number=w149) -> (double precision float=w148:dbl)
                n938 = Subtract(x=1.0, y=w152) -> (x-y=w150:dbl)
                n939 = To Double Precision Float(number=w146) -> (double precision float=w145:dbl)
                n940 = Multiply(x=w150, y=w148) -> (x*y=w147:dbl)
                n941 = Add(x=w147, y=w145) -> (x+y=w144:dbl)
                n942 = Round To Nearest(number=w144) -> (nearest integer value=w143:dbl)
                n943 = local read "left Coords"() -> (w157:T1)
                n944 = To Long Integer(number=w143) -> (32bit integer=w142:i32)
                n945 = Bundle By Name(cluster=w157, "Vertical"=w142) -> (w158:T1)
              }
            }
            n946 = local write "left Coords"(w109) -> ()
          }
          event "Line Profile": Value Change {
            n947 = event-data() -> ("NewVal"=w163:string)  [unwired: 1 in, 3 out]
            n948 = control-ref of="Left Graph"() -> (w164:refnum<vi>)
            n949 = case shown="\"Vertical\"" w163 {
              tunnel: w164 -> [_ w184]
              tunnel: w162 -> [w166 w179]
              tunnel: w161 -> [w165 w178]
              frame "Horizontal", Default {
                n950 = property on="left profie location" class="DigNum (strict)"("Precision"=w166, "Increment"=w165) -> ()  [unwired: 2 in, 2 out]
                n951 = property on="right wvf graph" class="WFGraph (strict)"() -> ("XScale.Multiplier"=w173:dbl, "XScale.Offset"=w174:dbl, "XScale.Maximum"=w175:dbl)  [unwired: 2 in, 2 out]
                n952 = property on="left wvf graph" class="WFGraph (strict)"("XScale.ScaleFit"=u8 1 ("X Scale.Scale Fit")) -> (error out=w170:errorcluster)  [unwired: 2 in, 1 out]
                n953 = property on="left wvf graph" class="WFGraph (strict)"(error in=w170, "XScale.Multiplier"=w173, "XScale.Offset"=w174, "XScale.Maximum"=w175, "XScale.NameLbl.Text"="Wavelength" ("X Scale.Name Label.Text")) -> ()  [unwired: 1 in, 2 out]
                n954 = property on="left Wavelength" class="DigNum (strict)"("Caption.Text"="Wavelength", "Increment"=1.0 ("Data Entry Limits:Increment"), "Precision"=u8 2 ("Display Format:Precision")) -> ()  [unwired: 2 in, 2 out]
              }
              frame "Vertical" {
                n955 = property on="left profie location" class="DigNum (strict)"("Precision"=u8 5 ("Display Format:Precision"), "Increment"=1.0 ("Data Entry Limits:Increment")) -> ()  [unwired: 2 in, 2 out]
                n956 = property on="Property Node" class="IntGraph (strict)"(reference=w184) -> ("YScale.Multiplier"=w185:dbl, "YScale.Offset"=w186:dbl, "YScale.Maximum"=w187:dbl)  [unwired: 1 in, 2 out]
                n957 = property on="left wvf graph" class="WFGraph (strict)"("XScale.ScaleFit"=u8 0 ("X Scale.Scale Fit")) -> (error out=w180:errorcluster)  [unwired: 2 in, 1 out]
                n958 = property on="left wvf graph" class="WFGraph (strict)"(error in=w180, "XScale.Multiplier"=w185, "XScale.Offset"=w186, "XScale.Maximum"=w187, "XScale.NameLbl.Text"="Y (mm)" ("X Scale.Name Label.Text")) -> ()  [unwired: 1 in, 2 out]
                n959 = property on="left Wavelength" class="DigNum (strict)"("Caption.Text"="Y (mm)", "Precision"=w179, "Increment"=w178) -> ()  [unwired: 2 in, 2 out]
              }
            }
          }
          event "left wvf scale 2": Value Change {
            n960 = event-data() -> ("NewVal"=w189:bool)  [unwired: 1 in, 5 out]
            n961 = case shown="True" w189 {
              tunnel: [0 2] -> w188
              frame False {
              }
              frame True {
              }
            }
            n962 = property on="left wvf graph" class="WFGraph (strict)"("YScale.ScaleFit"=w188) -> ()  [unwired: 2 in, 2 out]
          }
          event "right wvf scale 3": Value Change {
            n963 = event-data() -> ("NewVal"=w192:bool)  [unwired: 1 in, 5 out]
            n964 = case shown="True" w192 {
              tunnel: [0 2] -> w193
              frame False {
              }
              frame True {
              }
            }
            n965 = property on="right wvf graph" class="WFGraph (strict)"("YScale.ScaleFit"=w193) -> ()  [unwired: 2 in, 2 out]
          }
        }
        n966 = local read "Shut Down"() -> (w58:bool)
      }
    }
    frame #3 {
      # "for whatever reason the enum for open and close is reversed here"
      n967 = flat-sequence {
        frame #0 {
          n968 = call "stageGoAbs.vi"("abs pos"=0.0) -> ()  [unwired: 11 in]
        }
        frame #1 {
          n969 = global read "applicationControl.vi" "hasIxon"() -> (w1109:bool)
          n970 = case shown="True" w1109 {
            frame False {
            }
            frame True {
              n971 = in-place {
                n972 = call <userlib>:"CoolerOFF.vi"() -> ("error out"=w1110:errorcluster)  [unwired: 2 in, 1 out]
                n973 = call <userlib>:"SetShutter.vi"("type"=Shutter_type_typedef."TTL Low", "mode"=Shutter_mode_typedef."Open", "error in (no error)"=w1110) -> ()  [unwired: 11 in, 2 out]
                n974 = while {
                  stop <- w1114 stop-if-true
                  n975 = flat-sequence {
                    tunnel: [w1117] -> w1114
                    frame #0 {
                      n976 = call <userlib>:"GetTemperature.vi"() -> ("status"=w1115:T2, "temperature"=w1116:i32)  [unwired: 4 in, 2 out]
                      n977 = local write "Temperature"(w1116) -> ()
                      n978 = local write "temp. status 2"(w1115) -> ()
                      n979 = Greater Or Equal?(x=w1116, y=0) -> (x >= y?=w1117:bool)
                    }
                    frame #1 {
                      n980 = Wait (ms)(milliseconds to wait=u32 2000) -> ()  [unwired: 1 out]
                    }
                  }
                  n981 = Not(x=w1114) -> (.not. x?=→"Recovering Temperature":bool)
                }
              }
            }
          }
        }
        frame #2 {
          n982 = control-ref of="This VI"() -> (w1120:refnum<vi>)
          n983 = invoke class="VI" method="Default Vals.Reinit All"(reference=w1120) -> ()  [unwired: 2 in, 3 out]
          n984 = invoke on="Shut Down" class="Bool (strict)" method="Reinit To Default"() -> ()  [unwired: 3 in, 3 out]
        }
      }
    }
  }
